vi "Batched Execution Engine constants.vi"() -> ()   [LabVIEW 2010]
uses:
  <vilib>/addons/database/_DB Variant To Data/Database Variant To Data.xnode
  <vilib>/Utility/config.llb/Read Key (String).vi
  <vilib>/addons/database/Connection.llb/DB Tools Open Connec (String).vi
  <vilib>/addons/database/Connection.llb/Conn Execute.vi
  <vilib>/addons/database/Recordset.llb/Rec Destroy - Connection.vi
  <vilib>/addons/database/NI_Database_API.lvlib
  <vilib>/xml/NI_XML.lvlib
  <vilib>/Utility/VariantDataType/VariantType.lvlib
  <vilib>/Utility/config.llb/NI_LVConfig.lvlib
panel:
  out "error out 2":errorcluster
  out "Control Value:Get":variant
  out "error in (no error) 2":errorcluster
  out "submit_time":timestamp
  out "exec_time":timestamp
  in  "Parameter out":T1(array[cluster])
  out "error in (no error)":errorcluster
  out "exp_id":i32
  out "Result: XML Footer":string
  out "Result: XML Header":string
  out "Control TAG":string
  out "Indicator TAG":string
  out "Experiment VI":string
  out "Database":string
  out "CSG 2":csg caption="CSG"
  out "CDB 2":cdb caption="CDB"
  out "CXT 2":cxt caption="CXT"
  out "U 65":u64 caption="U 64"
  out "U 33":u32 caption="U 32"
  out "U 17":u16 caption="U 16"
  out "I 9":i64 caption="I 8"
  out "I 65":i64 caption="I 64"
  out "EXT 2":ext caption="EXT"
  out "I16 2":i16
  out "FXP 2":fxp<+,1,1> caption="FXP"
  out "Single 2":sgl
  out "I 33":i32 caption="I 32"
  out "U 9":i32 caption="U 8"
  out "String 2":string caption="String"
  out "Double 2":dbl caption="Double"
  in  "Parameter in":cluster{"parameter":string, "datatype":string}[](array[cluster])
  out "XML-String-out":string
  in  "input array":variant[](array[variant])
  out "output array":variant[](array[variant])
  out "parse errors":string
  in  "Write Status to Log file":bool
  out "XML-String-in":string
  in  "Stop":bool
  out "Status":string
  # "Parameter Tag"
  # "Parameter data type"
  # "Result Tag"
  # "Result Attribute"
  # "Settings"
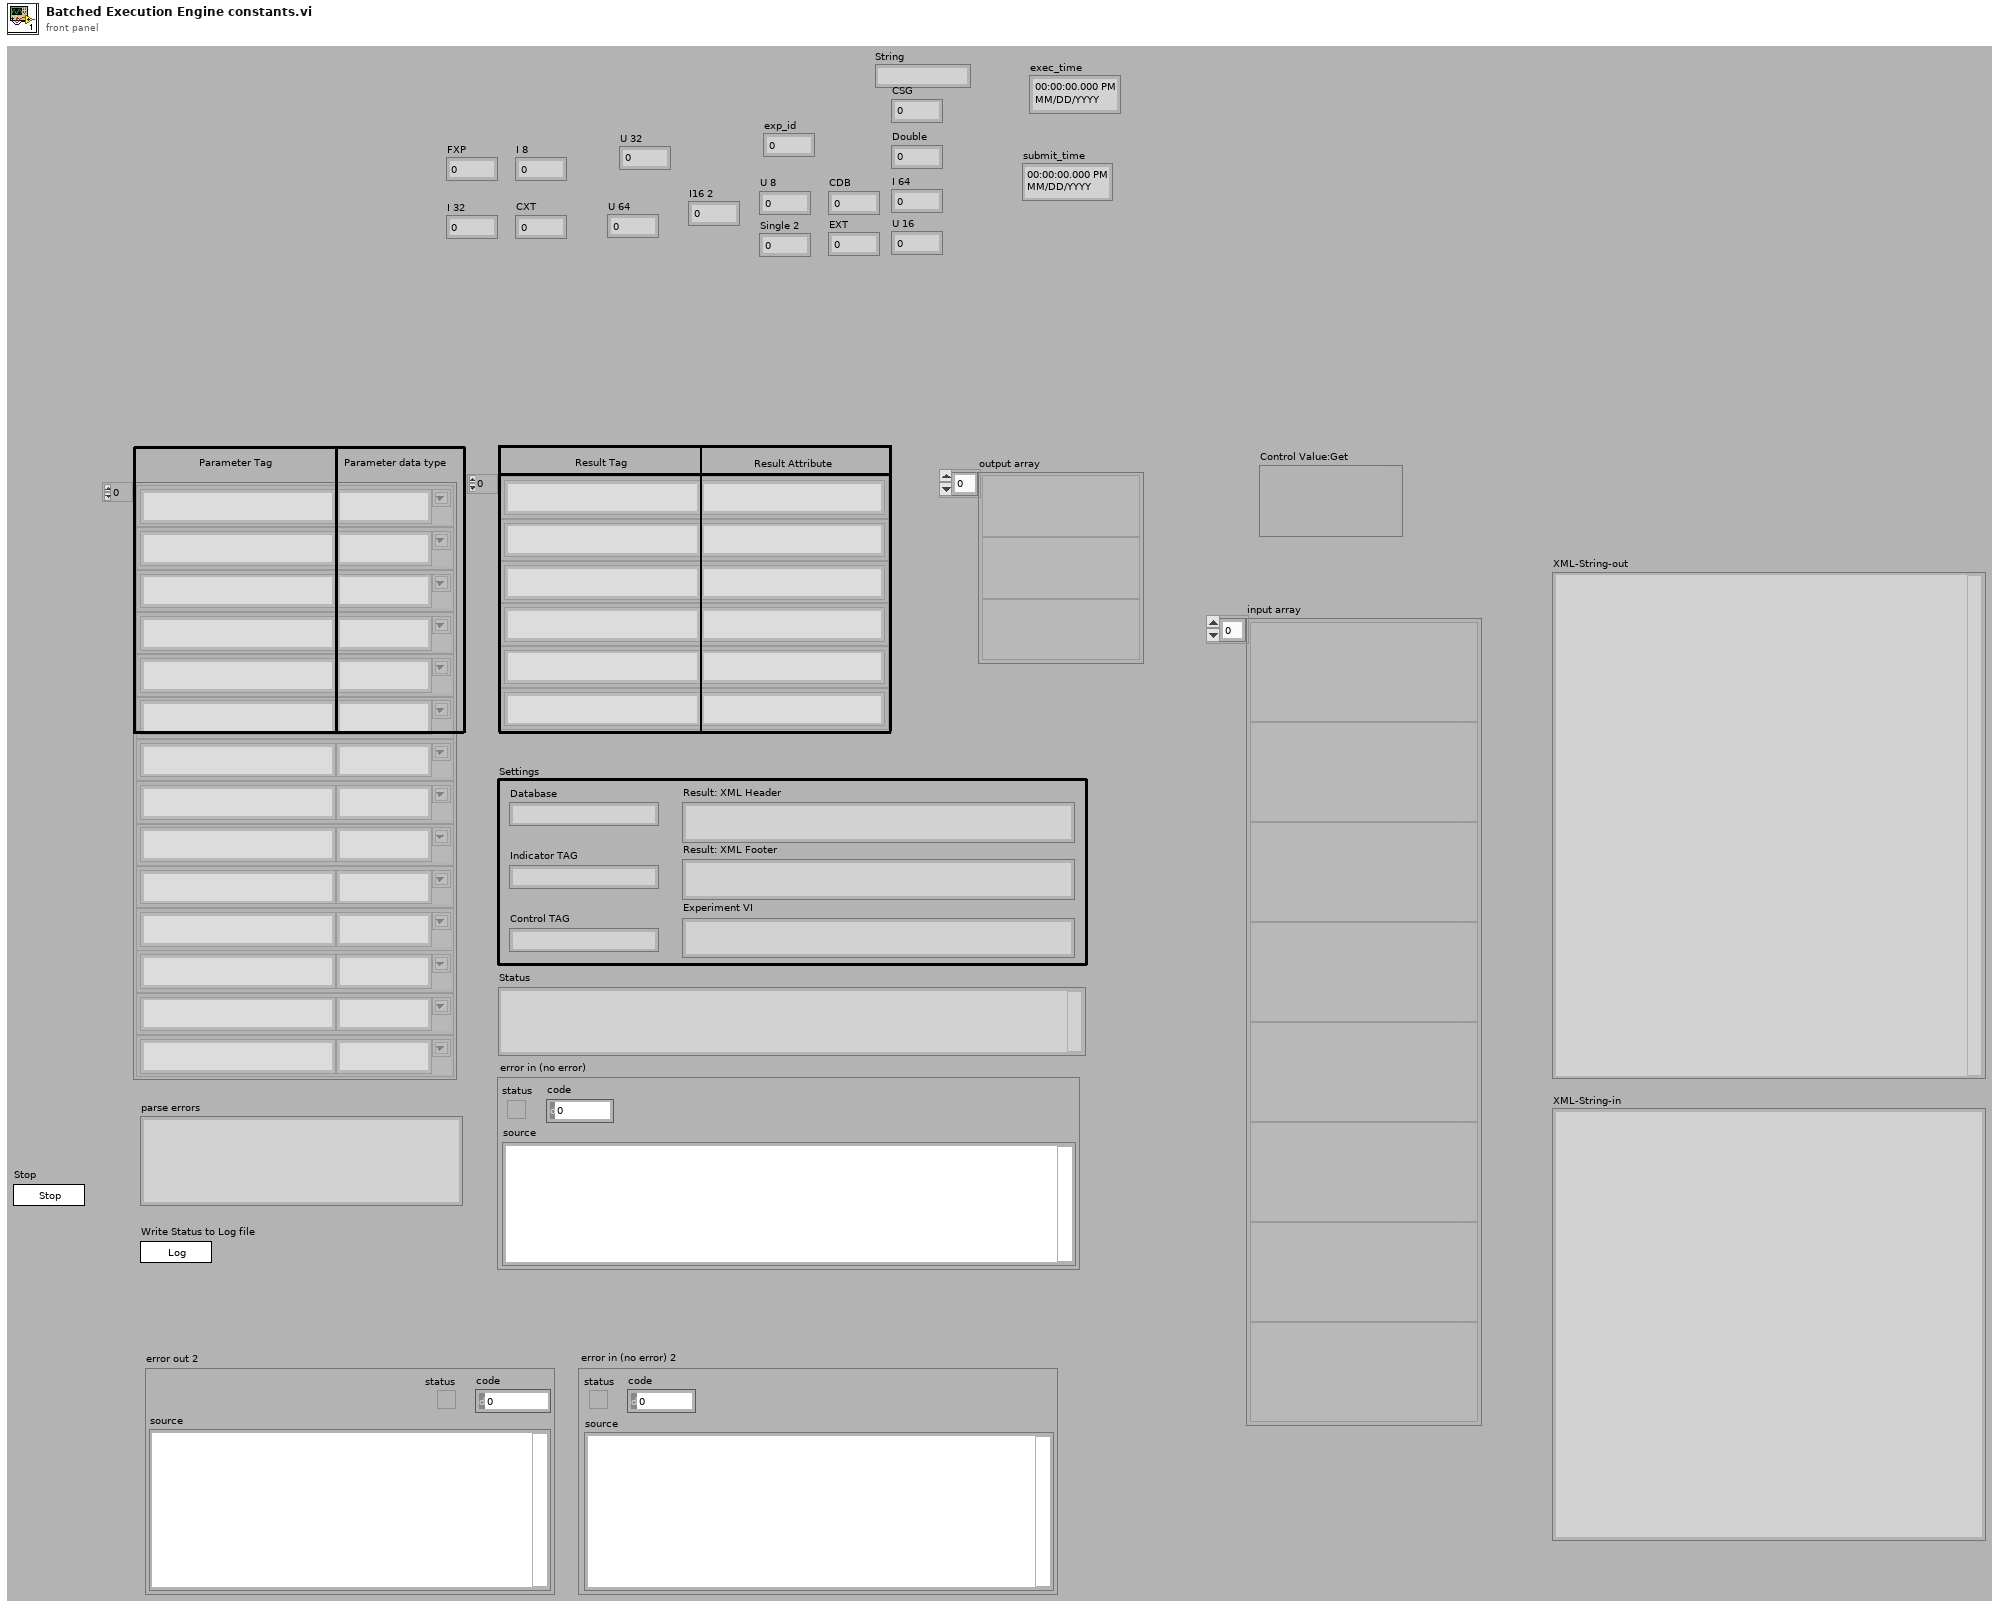
[diagram p1: front panel]
types:
  T1 = cluster{"parameter":string, "type info":string}[]
  T2 = enum16{"Search", "Parse", "Run", "Assemble", "Set", ""}
  T3 = typedef "NI_LVConfig.lvlib/Config Data RefNum.ctl" = refnum<k1>
  T4 = typedef "NI_Database_API.lvlib/Conn ObjectReference.ctl" = refnum<k1>
  T5 = typedef "NI_Database_API.lvlib/Rec ObjectReference.ctl" = refnum<k1>
  T6 = typedef "VariantType.lvlib/Type.ctl" = enum8{"Invalid Type", "Void", "I8", "I16", "I32", "I64", "U8", "U16", "U32", "U64", "Single Float", "Double Float", "Extended Float", "Single Complex", "Double Complex", "Extended Complex", "Enum U8", "Enum U16", "Enum U32", "Enum U64", "Single Float With Unit", "Double Float With Unit", "Extended Float With Unit", "Single Complex with Unit", "Double Complex with Unit", "Extended Complex with Unit", "Boolean", "String", "Path", "Picture", "Tag", "Array", "Cluster", "Variant", "LV Variant", "Waveform", "Timestamp", "Digital Waveform", "Digital Data", "ExpressData", "Refnum", "External Data", "VI", "Poly VI", "LabVIEW Class Instance", "Fixed Point"}
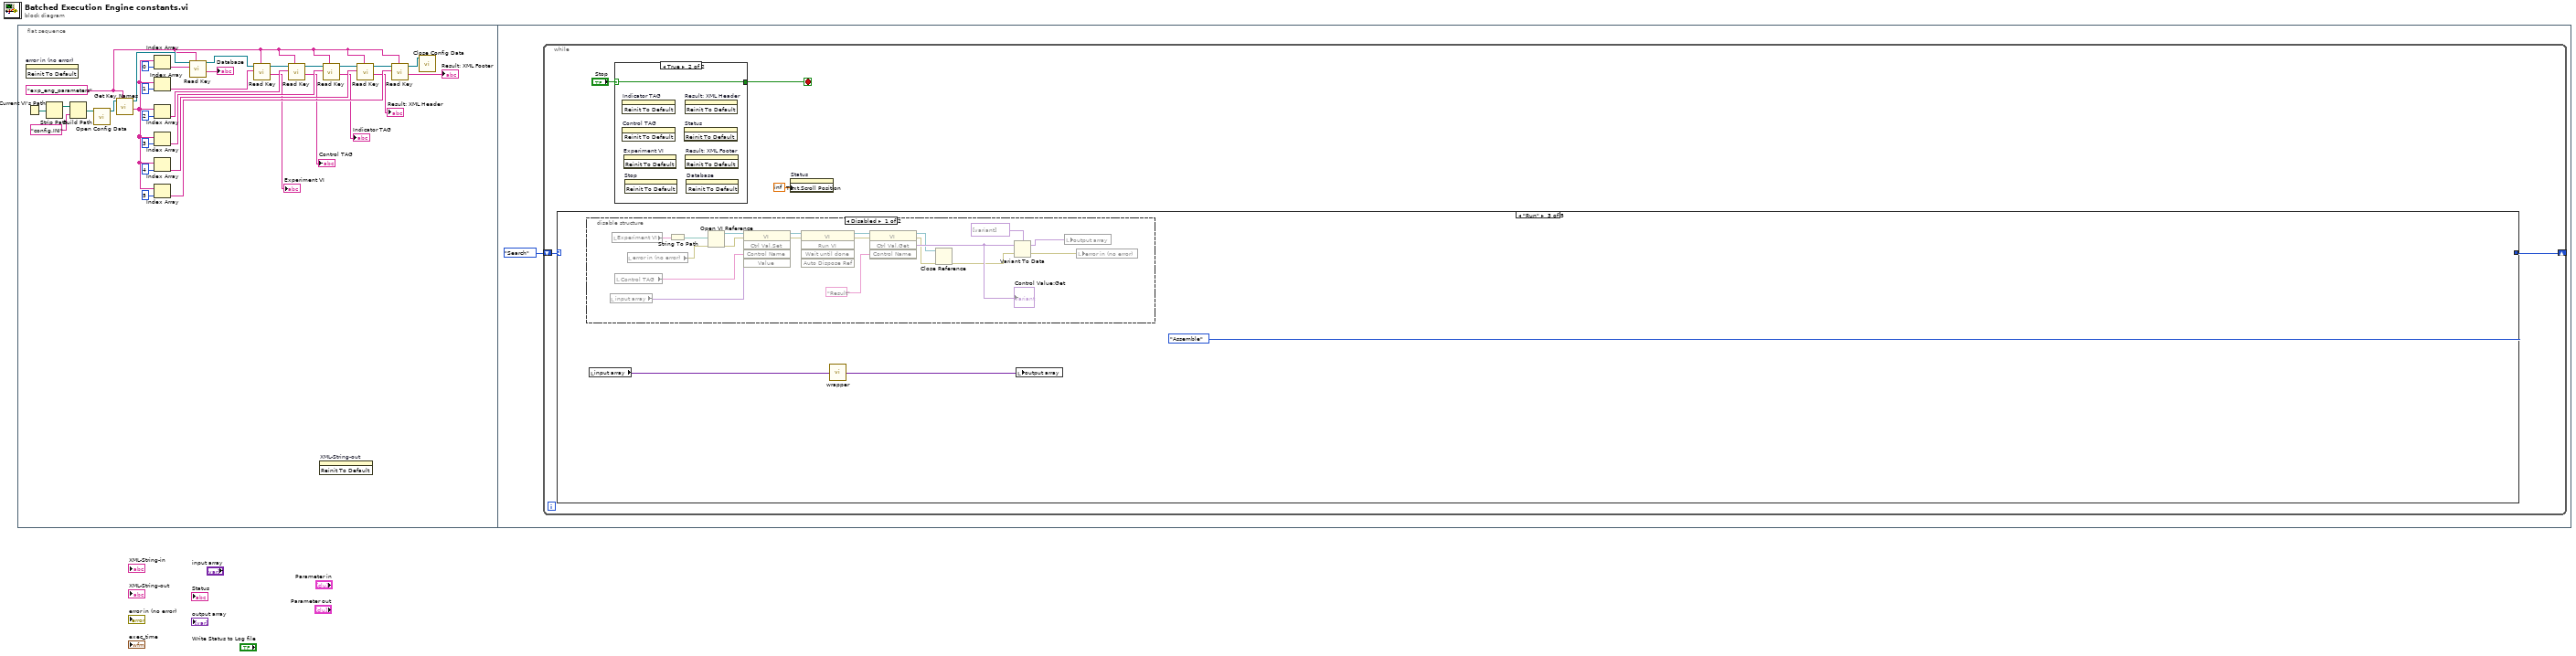
[diagram p0: block diagram]
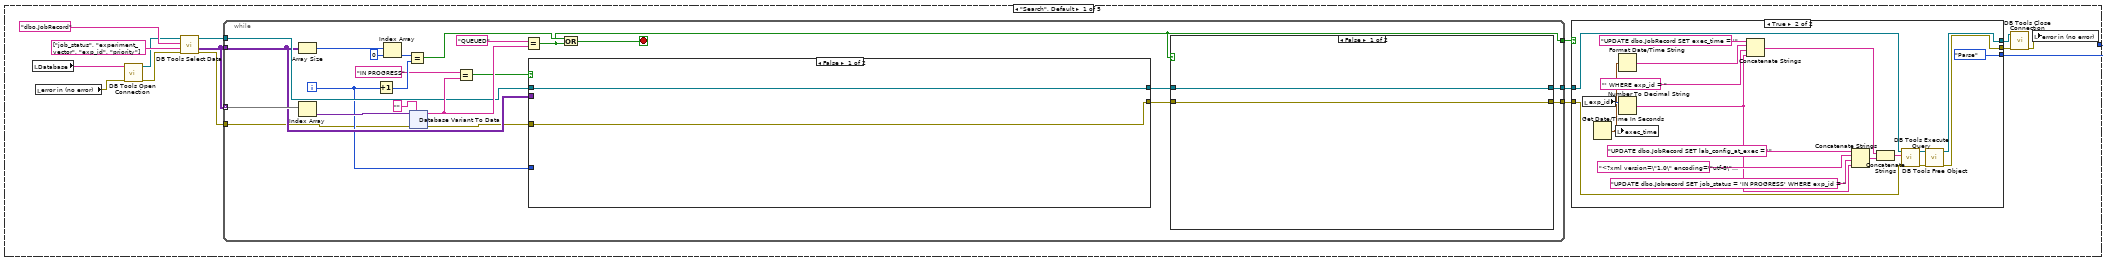
[diagram p3: hidden frame]
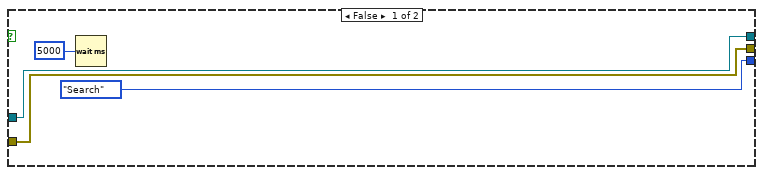
[diagram p4: hidden frame]
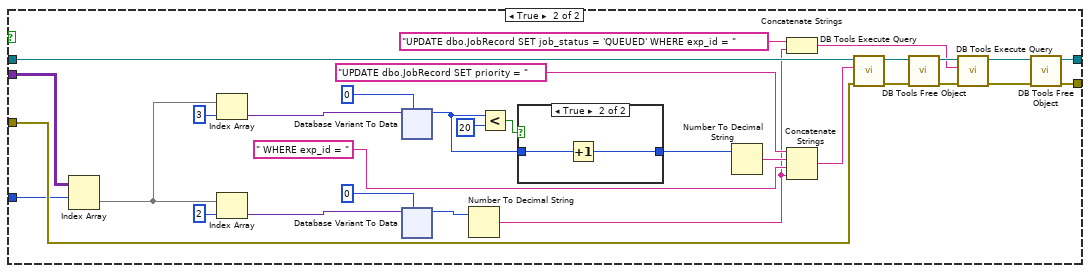
[diagram p5: hidden frame]
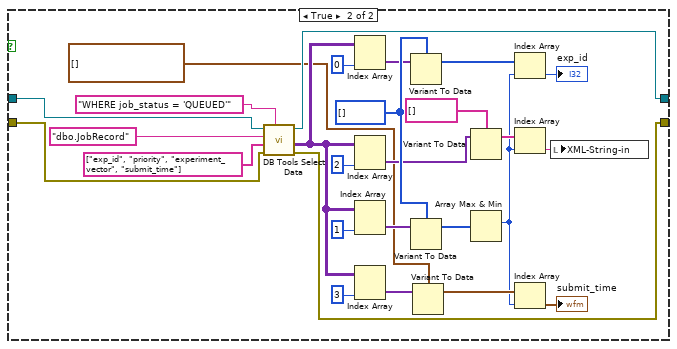
[diagram p7: hidden frame]
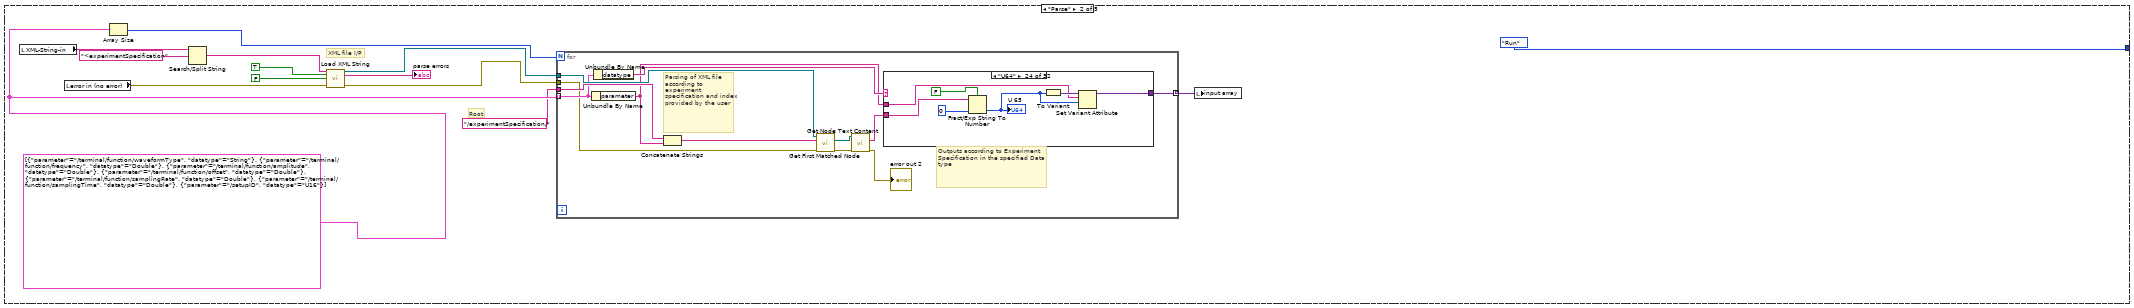
[diagram p8: hidden frame]
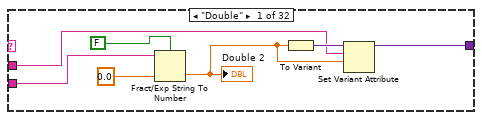
[diagram p9: hidden frame]
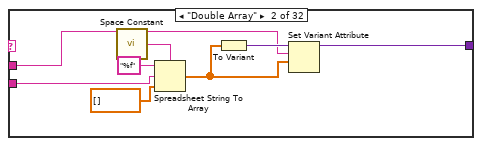
[diagram p10: hidden frame]
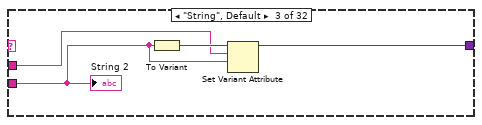
[diagram p11: hidden frame]
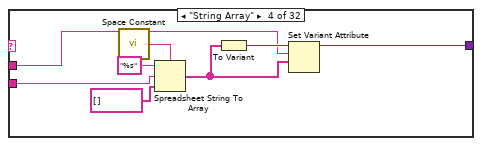
[diagram p12: hidden frame]
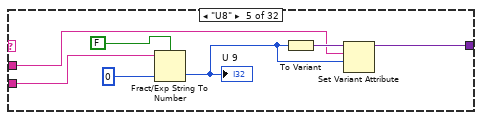
[diagram p13: hidden frame]
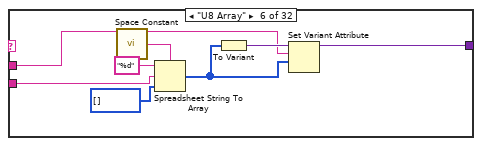
[diagram p14: hidden frame]
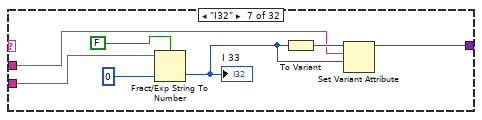
[diagram p15: hidden frame]
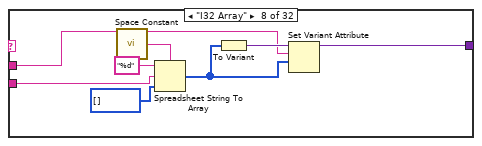
[diagram p16: hidden frame]
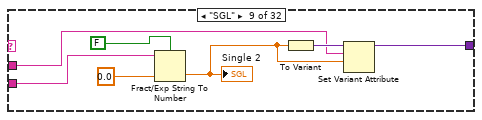
[diagram p17: hidden frame]
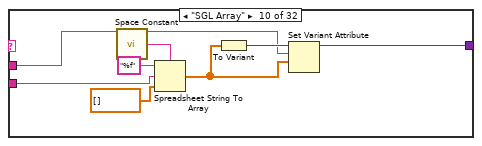
[diagram p18: hidden frame]
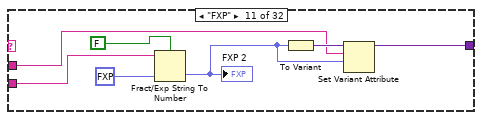
[diagram p19: hidden frame]
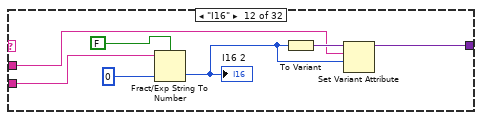
[diagram p20: hidden frame]
diagram:
  n1 = flat-sequence {
    frame #0 {
      w9 = "exp_eng_parameters" ("section")
      n2 = invoke on="error in (no error)" class="Clust (strict)" method="Reinit To Default"() -> ()  [unwired: 3 in, 3 out]
      n3 = Current VI's Path() -> (path=w32:path)
      n4 = Strip Path(path=w32) -> (stripped path=w31:path)  [unwired: 1 out]
      n5 = Build Path(base path=w31, name or relative path="config.INI") -> (appended path=w30:path)
      n6 = call <vilib>:"Open Config Data.vi"("configuration file path"=w30) -> ("refnum"=w28:T3)  [unwired: 8 in, 2 out]
      n7 = call <vilib>:"Get Key Names.vi"("section"=w9, "refnum"=w28) -> ("key names"=w11:string[], "refnum out"=w27:T3)  [unwired: 6 in, 2 out]
      n8 = Index Array(array=w11, index=0) -> (element=w25:string)
      n9 = Index Array(array=w11, index=1) -> (element=w23:string)
      n10 = Index Array(array=w11, index=2) -> (element=w19:string)
      n11 = Index Array(array=w11, index=3) -> (element=w16:string)
      n12 = Index Array(array=w11, index=4) -> (element=w14:string)
      n13 = Index Array(array=w11, index=5) -> (element=w10:string)
      n14 = call-poly <vilib>:"Read Key.vi"("section"=w9, "key"=w25, "refnum"=w27) -> ("value"=→"Database":string, "refnum out"=w22:T3)  [unwired: 5 in, 2 out]
      n15 = call-poly <vilib>:"Read Key.vi"("section"=w9, "key"=w23, "refnum"=w22) -> ("value"=→"Experiment VI":string, "refnum out"=w20:T3)  [unwired: 5 in, 2 out]
      n16 = call-poly <vilib>:"Read Key.vi"("section"=w9, "key"=w19, "refnum"=w20) -> ("value"=→"Control TAG":string, "refnum out"=w17:T3)  [unwired: 5 in, 2 out]
      n17 = invoke on="XML-String-out" class="Str" method="Reinit To Default"() -> ()  [unwired: 3 in, 3 out]
      n18 = call-poly <vilib>:"Read Key.vi"("section"=w9, "key"=w16, "refnum"=w17) -> ("value"=→"Indicator TAG":string, "refnum out"=w13:T3)  [unwired: 5 in, 2 out]
      n19 = call-poly <vilib>:"Read Key.vi"("section"=w9, "key"=w14, "refnum"=w13) -> ("value"=→"Result: XML Header":string, "refnum out"=w8:T3)  [unwired: 5 in, 2 out]
      n20 = call-poly <vilib>:"Read Key.vi"("section"=w9, "key"=w10, "refnum"=w8) -> ("value"=→"Result: XML Footer":string, "refnum out"=w7:T3)  [unwired: 5 in, 2 out]
      n21 = call <vilib>:"Close Config Data.vi"("refnum"=w7) -> ()  [unwired: 9 in, 2 out]
    }
    frame #1 {
      n22 = while {
        shift-right: [w37] -> _
        shift-left: T2."Search" -> [w38]
        stop <- w34 stop-if-true
        n23 = case shown="\"Run\"" w38 {
          tunnel: [w52 T2."Run" T2."Assemble" T2."Set" T2."Search"] -> w37
          frame "Search", Default {
            n24 = local read "Database"() -> (w51:string)
            n25 = local read "error in (no error)"() -> (w47:errorcluster)
            n26 = call-poly <vilib>:"DB Tools Open Connection.vi"("error in (no error)"=w47, "connection information"=w51) -> ("error out"=w54:errorcluster, "connection reference"=w42:T4)  [unwired: 6 in]
            n27 = call <vilib>:"DB Tools Select Data.vi"("error in (no error)"=w54, "columns"=string[] ["job_status", "experiment_vector", "exp_id", "priority"], "table"="dbo.JobRecord", "connection reference"=w42) -> ("error out"=w46:errorcluster, "data"=w53:variant[][], "connection reference out"=w41:T4)  [unwired: 2 in]
            n28 = while {
              tunnel: w41 -> [w90]
              tunnel: [w94] -> w50
              tunnel: w53 -> [w99] mode=indexing
              tunnel: w53 -> [w88]
              tunnel: [w85] -> w43
              tunnel: w46 -> [w81]
              tunnel: [w82] -> w45
              i -> [w87]
              stop <- w84 stop-if-true
              n29 = Array Size(array=w88) -> (size(s)=w98:i32[])
              n30 = Index Array(array=w99) -> (element=w100:variant)  [unwired: 1 in]
              n31 = Increment(x=w87) -> (x+1=w95:i32)
              n32 = Index Array(array=w98, index=0) -> (element=w96:i32)
              n33 = Equal?(x=w96, y=w95) -> (x = y?=w86:bool)
              n34 = xnode "Database Variant To Data"("database variant"=w100, "error in"=w81, "type"="") -> ("data"=w93:string, "error out"=w80:errorcluster)
              n35 = Equal?(x="IN PROGRESS", y=w93) -> (x = y?=w91:bool)
              n36 = Equal?(x="QUEUED", y=w93) -> (x = y?=w85:bool)
              n37 = case shown="False" w91 {
                tunnel: w90 -> [w104 w124]
                tunnel: [w104 w120] -> w89
                tunnel: w88 -> [_ w135]
                tunnel: w87 -> [_ w105]
                tunnel: w80 -> [w103 w111]
                tunnel: [w103 w107] -> w83
                frame False {
                }
                frame True {
                  n38 = Index Array(array=w135, index (row)=w105) -> (element=w128:variant[])  [unwired: 1 in]
                  n39 = Index Array(array=w128, index=3) -> (element=w133:variant)
                  n40 = Index Array(array=w128, index=2) -> (element=w126:variant)
                  n41 = xnode "Database Variant To Data"("database variant"=w133, "type"=0 ("index")) -> ("data"=w129:i32)  [unwired: 1 in, 1 out]
                  n42 = xnode "Database Variant To Data"("database variant"=w126, "type"=0 ("index")) -> ("data"=w115:i32)  [unwired: 1 in, 1 out]
                  n43 = Number To Decimal String(number=w115) -> (decimal integer string=w112:string)  [unwired: 1 in]
                  n44 = Less?(x=w129, y=20) -> (x < y?=w130:bool)
                  n45 = case shown="True" w130 {
                    tunnel: w129 -> [w168 w170]
                    tunnel: [w168 w169] -> w118
                    frame False {
                    }
                    frame True {
                      n46 = Increment(x=w170) -> (x+1=w169:i32)
                    }
                  }
                  n47 = Number To Decimal String(number=w118) -> (decimal integer string=w117:string)  [unwired: 1 in]
                  n48 = Concatenate Strings("UPDATE dbo.JobRecord SET job_status = 'QUEUED' WHERE exp_id = " ("string"), w112) -> (w106:string)
                  n49 = Concatenate Strings("UPDATE dbo.JobRecord SET priority = " ("string"), w117, " WHERE exp_id = " ("string"), w112) -> (w114:string)
                  n50 = call-poly <vilib>:"DB Tools Execute Query.vi"("error in (no error)"=w111, "SQL query"=w114, "connection reference"=w124) -> ("error out"=w110:errorcluster, "recordset reference"=w123:T5)  [unwired: 5 in]
                  n51 = call-poly <vilib>:"DB Tools Free Object.vi"("error in (no error)"=w110, "recordset reference"=w123) -> ("error out"=w109:errorcluster, "connection reference"=w122:T4)  [unwired: 8 in]
                  n52 = call-poly <vilib>:"DB Tools Execute Query.vi"("error in (no error)"=w109, "SQL query"=w106, "connection reference"=w122) -> ("error out"=w108:errorcluster, "recordset reference"=w121:T5)  [unwired: 5 in]
                  n53 = call-poly <vilib>:"DB Tools Free Object.vi"("error in (no error)"=w108, "recordset reference"=w121) -> ("error out"=w107:errorcluster, "connection reference"=w120:T4)  [unwired: 8 in]
                }
              }
              n54 = Or(x=w86, y=w85) -> (x .or. y?=w84:bool)
              n55 = case shown="False" w85 {
                tunnel: w89 -> [w236 w254]
                tunnel: [w236 w253] -> w94
                tunnel: w83 -> [w235 w248]
                tunnel: [w235 w247] -> w82
                frame False {
                }
                frame True {
                  w261 = i32[] [] ("Array")
                  n56 = call <vilib>:"DB Tools Select Data.vi"("condition"="WHERE job_status = 'QUEUED'" ("optional clause"), "error in (no error)"=w248, "columns"=string[] ["exp_id", "priority", "experiment_vector", "submit_time"], "table"="dbo.JobRecord", "connection reference"=w254) -> ("error out"=w247:errorcluster, "data"=w243:variant[][], "connection reference out"=w253:T4)  [unwired: 1 in]
                  n57 = Index Array(array=w243, index (col)=0 ("disabled index (col)")) -> (element=w260:variant[])  [unwired: 1 in]
                  n58 = Index Array(array=w243, index (col)=2 ("index (row)")) -> (element=w251:variant[])  [unwired: 1 in]
                  n59 = Index Array(array=w243, index (col)=1 ("disabled index (col)")) -> (element=w258:variant[])  [unwired: 1 in]
                  n60 = Index Array(array=w243, index (col)=3 ("disabled index (col)")) -> (element=w241:variant[])  [unwired: 1 in]
                  n61 = Variant To Data(Variant=w260, type=w261) -> (data=w263:i32[])  [unwired: 1 in, 1 out]
                  n62 = Variant To Data(Variant=w258, type=w261) -> (data=w262:i32[])  [unwired: 1 in, 1 out]
                  n63 = Variant To Data(Variant=w241, type=timestamp[] [] ("Array")) -> (data=w239:timestamp[])  [unwired: 1 in, 1 out]
                  n64 = Variant To Data(Variant=w251, type=string[] [] ("Array")) -> (data=w250:string[])  [unwired: 1 in, 1 out]
                  n65 = Array Max & Min(array=w262) -> (max index (indices)=w238:i32)  [unwired: 3 out]
                  n66 = Index Array(array=w263, index=w238) -> (element=→"exp_id":i32)
                  n67 = Index Array(array=w250, index=w238) -> (element=w249:string)
                  n68 = Index Array(array=w239, index=w238) -> (element=→"submit_time":timestamp)
                  n69 = local write "XML-String-in"(w249) -> ()
                }
              }
            }
            n70 = case shown="True" w43 {
              tunnel: [T2."Search" T2."Parse"] -> w52
              tunnel: [w60 w72] -> w49
              tunnel: w50 -> [w60 w78]
              tunnel: w45 -> [w59 w77]
              tunnel: [w59 w75] -> w48
              frame False {
                n71 = Wait (ms)(milliseconds to wait=u32 5000 ("millisecond multiple")) -> ()  [unwired: 1 out]
              }
              frame True {
                n72 = local read "exp_id"() -> (w74:i32)
                n73 = Get Date/Time In Seconds() -> (seconds since 1Jan1904=w61:timestamp)
                n74 = local write "exec_time"(w61) -> ()
                n75 = Format Date/Time String(seconds (now)=w61) -> (date/time string=w70:string)  [unwired: 2 in]
                n76 = Number To Decimal String(number=w74) -> (decimal integer string=w65:string)  [unwired: 1 in]
                n77 = Concatenate Strings("UPDATE dbo.JobRecord SET exec_time = '", w70, "' WHERE exp_id = ", w65) -> (w64:string)
                n78 = Concatenate Strings("UPDATE dbo.JobRecord SET lab_config_at_exec = '" ("string"), "<?xml version=\"1.0\" encoding=\"utf-8\" standalone=\"no\" ?><!DOCTYPE labConfiguration SYSTEM \"http://web.mit.edu/weblab/xml/labConfiguration.dtd\"><labConfiguration lab=\"MIT ELVIS Weblab\" specversion=\"0.1\">'" ("string"), "UPDATE dbo.Jobrecord SET job_status = 'IN PROGRESS' WHERE exp_id = " ("string"), w65) -> (w63:string)
                n79 = Concatenate Strings(w64, w63) -> (w62:string)
                n80 = call-poly <vilib>:"DB Tools Execute Query.vi"("error in (no error)"=w77, "SQL query"=w62, "connection reference"=w78) -> ("error out"=w76:errorcluster, "recordset reference"=w73:T5)  [unwired: 5 in]
                n81 = call-poly <vilib>:"DB Tools Free Object.vi"("error in (no error)"=w76, "recordset reference"=w73) -> ("error out"=w75:errorcluster, "connection reference"=w72:T4)  [unwired: 8 in]
              }
            }
            n82 = call <vilib>:"DB Tools Close Connection.vi"("error in (no error)"=w48, "connection reference"=w49) -> ("error out"=w44:errorcluster)  [unwired: 5 in]
            n83 = local write "error in (no error)"(w44) -> ()
          }
          frame "Parse" {
            w265 = cluster{"parameter":string, "datatype":string}[] [{"parameter"="/terminal/function/waveformType", "datatype"="String"}, {"parameter"="/terminal/function/frequency", "datatype"="Double"}, {"parameter"="/terminal/function/amplitude", "datatype"="Double"}, {"parameter"="/terminal/function/offset", "datatype"="Double"}, {"parameter"="/terminal/function/samplingRate", "datatype"="Double"}, {"parameter"="/terminal/function/samplingTime", "datatype"="Double"}, {"parameter"="/setupID", "datatype"="U16"}]
            # "Root"
            # "XML file I/P"
            n84 = local read "XML-String-in"() -> (w270:string)
            n85 = local read "error in (no error)"() -> (w271:errorcluster)
            n86 = Array Size(array=w265) -> (size(s)=w267:i32)
            n87 = Search/Split String(string=w270, search string/char (-)="<experimentSpecification") -> (match + rest of string=w268:string)  [unwired: 1 in, 2 out]
            n88 = call <vilib>:"Load XML String.vi"("XML string"=w268, "process namespaces (False)"=TRUE, "process schema (False)"=FALSE, "error in (no error)"=w271) -> ("DOM document out"=w273:refnum<k20>, "parse errors"=→"parse errors":string, "error out"=w266:errorcluster)  [unwired: 9 out]
            n89 = for {
              N: w267 -> [_]
              tunnel: w273 -> [w289]
              tunnel: "/experimentSpecification/" -> [w287]
              tunnel: w265 -> [w285] mode=indexing
              tunnel: w266 -> [w284]
              tunnel: [w283] -> w272 mode=indexing
              # "Outputs according to Experiment Specification in the specified Data type"
              # "Parsing of XML file according to experiment specification and index provided by the user"
              n90 = Unbundle By Name(w285) -> ("parameter"=w280:string)
              n91 = Unbundle By Name(w285) -> ("datatype"=w282:string)
              n92 = Concatenate Strings(w287, w280) -> (w286:string)
              n93 = call <vilib>:"Get First Matched Node.vi"("error in (no error)"=w284, "XPath expression"=w286, "node in"=w289) -> ("error out"=w278:errorcluster, "node result"=w288:refnum<k20>)  [unwired: 6 in, 1 out]
              n94 = call <vilib>:"Get Node Text Content.vi"("error in (no error)"=w278, "node in"=w288) -> ("error out"=→"error out 2":errorcluster, "node text"=w281:string)  [unwired: 7 in, 1 out]
              n95 = case shown="\"U64\"" w282 {
                tunnel: w280 -> [w290 w298 w305 w309 w317 w324 w332 w340 w347 w355 w362 w369 w376 w384 w392 w399 w406 w414 w421 w429 w436 w444 w451 w459 w466 w474 w482 w490 w497 w504 w512 w519]
                tunnel: w281 -> [w291 w297 w306 w310 w318 w325 w333 w339 w348 w354 w363 w370 w377 w385 w391 w400 w407 w415 w422 w430 w437 w445 w452 w460 w467 w475 w481 w489 w496 w505 w511 w520]
                tunnel: [w293 w300 w307 w313 w320 w328 w335 w343 w350 w357 w365 w372 w380 w387 w394 w402 w410 w417 w425 w432 w440 w447 w455 w462 w470 w477 w484 w492 w499 w507 w514 w522] -> w283
                frame "Double" {
                  n96 = Fract/Exp String To Number(use system decimal point (T)=FALSE, string=w291, default (0 dbl)=0.0) -> (number=w292:dbl)  [unwired: 1 in, 1 out]
                  "Double 2" <- w292
                  n97 = To Variant(anything=w292) -> (Variant=w294:variant)
                  n98 = Set Variant Attribute(Variant=w294, name=w290, value=w292) -> (Variant out=w293:variant)  [unwired: 1 in, 2 out]
                }
                frame "Double Array" {
                  n99 = call <vilib>:"Space Constant.vi"() -> ("String"=w302:string)
                  n100 = Spreadsheet String To Array(delimiter (Tab)=w302, format string="%f", spreadsheet string=w297, array type (2D Dbl)=dbl[] [] ("Array")) -> (array=w299:dbl[])
                  n101 = To Variant(anything=w299) -> (Variant=w301:variant)
                  n102 = Set Variant Attribute(Variant=w301, name=w298, value=w299) -> (Variant out=w300:variant)  [unwired: 1 in, 2 out]
                }
                frame "String", Default {
                  n103 = To Variant(anything=w306) -> (Variant=w308:variant)
                  n104 = Set Variant Attribute(Variant=w308, name=w305, value=w306) -> (Variant out=w307:variant)  [unwired: 1 in, 2 out]
                  "String 2" <- w306
                }
                frame "String Array" {
                  n105 = call <vilib>:"Space Constant.vi"() -> ("String"=w315:string)
                  n106 = Spreadsheet String To Array(delimiter (Tab)=w315, format string="%s", spreadsheet string=w310, array type (2D Dbl)=string[] [] ("Array")) -> (array=w312:string[])
                  n107 = To Variant(anything=w312) -> (Variant=w314:variant)
                  n108 = Set Variant Attribute(Variant=w314, name=w309, value=w312) -> (Variant out=w313:variant)  [unwired: 1 in, 2 out]
                }
                frame "U8" {
                  n109 = Fract/Exp String To Number(use system decimal point (T)=FALSE, string=w318, default (0 dbl)=u8 0) -> (number=w319:u8)  [unwired: 1 in, 1 out]
                  "U 9" <- w319
                  n110 = To Variant(anything=w319) -> (Variant=w321:variant)
                  n111 = Set Variant Attribute(Variant=w321, name=w317, value=w319) -> (Variant out=w320:variant)  [unwired: 1 in, 2 out]
                }
                frame "U8 Array" {
                  n112 = call <vilib>:"Space Constant.vi"() -> ("String"=w330:string)
                  n113 = Spreadsheet String To Array(delimiter (Tab)=w330, format string="%d", spreadsheet string=w325, array type (2D Dbl)=u8[] [] ("Array")) -> (array=w326:u8[])
                  n114 = To Variant(anything=w326) -> (Variant=w329:variant)
                  n115 = Set Variant Attribute(Variant=w329, name=w324, value=w326) -> (Variant out=w328:variant)  [unwired: 1 in, 2 out]
                }
                frame "I32" {
                  n116 = Fract/Exp String To Number(use system decimal point (T)=FALSE, string=w333, default (0 dbl)=0) -> (number=w334:i32)  [unwired: 1 in, 1 out]
                  "I 33" <- w334
                  n117 = To Variant(anything=w334) -> (Variant=w336:variant)
                  n118 = Set Variant Attribute(Variant=w336, name=w332, value=w334) -> (Variant out=w335:variant)  [unwired: 1 in, 2 out]
                }
                frame "I32 Array" {
                  n119 = call <vilib>:"Space Constant.vi"() -> ("String"=w345:string)
                  n120 = Spreadsheet String To Array(delimiter (Tab)=w345, format string="%d", spreadsheet string=w339, array type (2D Dbl)=i32[] [] ("Array")) -> (array=w341:i32[])
                  n121 = To Variant(anything=w341) -> (Variant=w344:variant)
                  n122 = Set Variant Attribute(Variant=w344, name=w340, value=w341) -> (Variant out=w343:variant)  [unwired: 1 in, 2 out]
                }
                frame "SGL" {
                  n123 = Fract/Exp String To Number(use system decimal point (T)=FALSE, string=w348, default (0 dbl)=sgl 0.0) -> (number=w349:sgl)  [unwired: 1 in, 1 out]
                  "Single 2" <- w349
                  n124 = To Variant(anything=w349) -> (Variant=w351:variant)
                  n125 = Set Variant Attribute(Variant=w351, name=w347, value=w349) -> (Variant out=w350:variant)  [unwired: 1 in, 2 out]
                }
                frame "SGL Array" {
                  n126 = call <vilib>:"Space Constant.vi"() -> ("String"=w359:string)
                  n127 = Spreadsheet String To Array(delimiter (Tab)=w359, format string="%f", spreadsheet string=w354, array type (2D Dbl)=sgl[] [] ("Array")) -> (array=w356:sgl[])
                  n128 = To Variant(anything=w356) -> (Variant=w358:variant)
                  n129 = Set Variant Attribute(Variant=w358, name=w355, value=w356) -> (Variant out=w357:variant)  [unwired: 1 in, 2 out]
                }
                frame "FXP" {
                  n130 = Fract/Exp String To Number(use system decimal point (T)=FALSE, string=w363, default (0 dbl)=fxp<+,1,1> 0.0) -> (number=w364:fxp<+,1,1>)  [unwired: 1 in, 1 out]
                  "FXP 2" <- w364
                  n131 = To Variant(anything=w364) -> (Variant=w366:variant)
                  n132 = Set Variant Attribute(Variant=w366, name=w362, value=w364) -> (Variant out=w365:variant)  [unwired: 1 in, 2 out]
                }
                frame "I16" {
                  n133 = Fract/Exp String To Number(use system decimal point (T)=FALSE, string=w370, default (0 dbl)=i16 0 ("I16")) -> (number=w373:i16)  [unwired: 1 in, 1 out]
                  "I16 2" <- w373
                  n134 = To Variant(anything=w373) -> (Variant=w374:variant)
                  n135 = Set Variant Attribute(Variant=w374, name=w369, value=w373) -> (Variant out=w372:variant)  [unwired: 1 in, 2 out]
                }
                frame "I16 Array" {
                  n136 = call <vilib>:"Space Constant.vi"() -> ("String"=w382:string)
                  n137 = Spreadsheet String To Array(delimiter (Tab)=w382, format string="%d", spreadsheet string=w377, array type (2D Dbl)=i16[] [] ("Array")) -> (array=w378:i16[])
                  n138 = To Variant(anything=w378) -> (Variant=w381:variant)
                  n139 = Set Variant Attribute(Variant=w381, name=w376, value=w378) -> (Variant out=w380:variant)  [unwired: 1 in, 2 out]
                }
                frame "EXT" {
                  n140 = Fract/Exp String To Number(use system decimal point (T)=FALSE, string=w385, default (0 dbl)=ext 0.0) -> (number=w386:ext)  [unwired: 1 in, 1 out]
                  "EXT 2" <- w386
                  n141 = To Variant(anything=w386) -> (Variant=w388:variant)
                  n142 = Set Variant Attribute(Variant=w388, name=w384, value=w386) -> (Variant out=w387:variant)  [unwired: 1 in, 2 out]
                }
                frame "EXT Array" {
                  n143 = call <vilib>:"Space Constant.vi"() -> ("String"=w396:string)
                  n144 = Spreadsheet String To Array(delimiter (Tab)=w396, format string="%f", spreadsheet string=w391, array type (2D Dbl)=ext[] [] ("Array")) -> (array=w393:ext[])
                  n145 = To Variant(anything=w393) -> (Variant=w395:variant)
                  n146 = Set Variant Attribute(Variant=w395, name=w392, value=w393) -> (Variant out=w394:variant)  [unwired: 1 in, 2 out]
                }
                frame "I64" {
                  n147 = Fract/Exp String To Number(use system decimal point (T)=FALSE, string=w400, default (0 dbl)=i64 0) -> (number=w401:i64)  [unwired: 1 in, 1 out]
                  "I 65" <- w401
                  n148 = To Variant(anything=w401) -> (Variant=w403:variant)
                  n149 = Set Variant Attribute(Variant=w403, name=w399, value=w401) -> (Variant out=w402:variant)  [unwired: 1 in, 2 out]
                }
                frame "I64 Array" {
                  n150 = call <vilib>:"Space Constant.vi"() -> ("String"=w412:string)
                  n151 = Spreadsheet String To Array(delimiter (Tab)=w412, format string="%d", spreadsheet string=w407, array type (2D Dbl)=i64[] [] ("Array")) -> (array=w408:i64[])
                  n152 = To Variant(anything=w408) -> (Variant=w411:variant)
                  n153 = Set Variant Attribute(Variant=w411, name=w406, value=w408) -> (Variant out=w410:variant)  [unwired: 1 in, 2 out]
                }
                frame "I8" {
                  n154 = Fract/Exp String To Number(use system decimal point (T)=FALSE, string=w415, default (0 dbl)=i8 0) -> (number=w416:i8)  [unwired: 1 in, 1 out]
                  "I 9" <- w416
                  n155 = To Variant(anything=w416) -> (Variant=w418:variant)
                  n156 = Set Variant Attribute(Variant=w418, name=w414, value=w416) -> (Variant out=w417:variant)  [unwired: 1 in, 2 out]
                }
                frame "I8 Array" {
                  n157 = call <vilib>:"Space Constant.vi"() -> ("String"=w427:string)
                  n158 = Spreadsheet String To Array(delimiter (Tab)=w427, format string="%d", spreadsheet string=w422, array type (2D Dbl)=i8[] [] ("Array")) -> (array=w423:i8[])
                  n159 = To Variant(anything=w423) -> (Variant=w426:variant)
                  n160 = Set Variant Attribute(Variant=w426, name=w421, value=w423) -> (Variant out=w425:variant)  [unwired: 1 in, 2 out]
                }
                frame "U16" {
                  n161 = Fract/Exp String To Number(use system decimal point (T)=FALSE, string=w430, default (0 dbl)=u16 0) -> (number=w431:u16)  [unwired: 1 in, 1 out]
                  "U 17" <- w431
                  n162 = To Variant(anything=w431) -> (Variant=w433:variant)
                  n163 = Set Variant Attribute(Variant=w433, name=w429, value=w431) -> (Variant out=w432:variant)  [unwired: 1 in, 2 out]
                }
                frame "U16 Array" {
                  n164 = call <vilib>:"Space Constant.vi"() -> ("String"=w442:string)
                  n165 = Spreadsheet String To Array(delimiter (Tab)=w442, format string="%d", spreadsheet string=w437, array type (2D Dbl)=u16[] [] ("Array")) -> (array=w438:u16[])
                  n166 = To Variant(anything=w438) -> (Variant=w441:variant)
                  n167 = Set Variant Attribute(Variant=w441, name=w436, value=w438) -> (Variant out=w440:variant)  [unwired: 1 in, 2 out]
                }
                frame "U32" {
                  n168 = Fract/Exp String To Number(use system decimal point (T)=FALSE, string=w445, default (0 dbl)=u32 0) -> (number=w446:u32)  [unwired: 1 in, 1 out]
                  "U 33" <- w446
                  n169 = To Variant(anything=w446) -> (Variant=w448:variant)
                  n170 = Set Variant Attribute(Variant=w448, name=w444, value=w446) -> (Variant out=w447:variant)  [unwired: 1 in, 2 out]
                }
                frame "U32 Array" {
                  n171 = call <vilib>:"Space Constant.vi"() -> ("String"=w457:string)
                  n172 = Spreadsheet String To Array(delimiter (Tab)=w457, format string="%d", spreadsheet string=w452, array type (2D Dbl)=u32[] [] ("Array")) -> (array=w453:u32[])
                  n173 = To Variant(anything=w453) -> (Variant=w456:variant)
                  n174 = Set Variant Attribute(Variant=w456, name=w451, value=w453) -> (Variant out=w455:variant)  [unwired: 1 in, 2 out]
                }
                frame "U64" {
                  n175 = Fract/Exp String To Number(use system decimal point (T)=FALSE, string=w460, default (0 dbl)=u64 0) -> (number=w461:u64)  [unwired: 1 in, 1 out]
                  "U 65" <- w461
                  n176 = To Variant(anything=w461) -> (Variant=w463:variant)
                  n177 = Set Variant Attribute(Variant=w463, name=w459, value=w461) -> (Variant out=w462:variant)  [unwired: 1 in, 2 out]
                }
                frame "U64 Array" {
                  n178 = call <vilib>:"Space Constant.vi"() -> ("String"=w472:string)
                  n179 = Spreadsheet String To Array(delimiter (Tab)=w472, format string="%d", spreadsheet string=w467, array type (2D Dbl)=u64[] [] ("Array")) -> (array=w468:u64[])
                  n180 = To Variant(anything=w468) -> (Variant=w471:variant)
                  n181 = Set Variant Attribute(Variant=w471, name=w466, value=w468) -> (Variant out=w470:variant)  [unwired: 1 in, 2 out]
                }
                frame "CXT" {
                  n182 = Scan From String(format string="%f", input string=w475, default 1=cxt 0.0+0.0i ("number 3")) -> (output 1=w476:cxt)  [unwired: 2 in, 3 out]
                  "CXT 2" <- w476
                  n183 = To Variant(anything=w476) -> (Variant=w478:variant)
                  n184 = Set Variant Attribute(Variant=w478, name=w474, value=w476) -> (Variant out=w477:variant)  [unwired: 1 in, 2 out]
                }
                frame "CXT Array" {
                  n185 = call <vilib>:"Space Constant.vi"() -> ("String"=w486:string)
                  n186 = Spreadsheet String To Array(delimiter (Tab)=w486, format string="%f", spreadsheet string=w481, array type (2D Dbl)=cxt[] [] ("Array")) -> (array=w483:cxt[])
                  n187 = To Variant(anything=w483) -> (Variant=w485:variant)
                  n188 = Set Variant Attribute(Variant=w485, name=w482, value=w483) -> (Variant out=w484:variant)  [unwired: 1 in, 2 out]
                }
                frame "CDB" {
                  n189 = Scan From String(format string="%f", input string=w489, default 1=cdb 0.0+0.0i ("number 3")) -> (output 1=w491:cdb)  [unwired: 2 in, 3 out]
                  "CDB 2" <- w491
                  n190 = To Variant(anything=w491) -> (Variant=w493:variant)
                  n191 = Set Variant Attribute(Variant=w493, name=w490, value=w491) -> (Variant out=w492:variant)  [unwired: 1 in, 2 out]
                }
                frame "CDB Array" {
                  n192 = call <vilib>:"Space Constant.vi"() -> ("String"=w501:string)
                  n193 = Spreadsheet String To Array(delimiter (Tab)=w501, format string="%f", spreadsheet string=w496, array type (2D Dbl)=cdb[] [] ("Array")) -> (array=w498:cdb[])
                  n194 = To Variant(anything=w498) -> (Variant=w500:variant)
                  n195 = Set Variant Attribute(Variant=w500, name=w497, value=w498) -> (Variant out=w499:variant)  [unwired: 1 in, 2 out]
                }
                frame "CSG" {
                  n196 = Scan From String(format string="%f", input string=w505, default 1=csg 0.0+0.0i ("number 3")) -> (output 1=w506:csg)  [unwired: 2 in, 3 out]
                  "CSG 2" <- w506
                  n197 = To Variant(anything=w506) -> (Variant=w508:variant)
                  n198 = Set Variant Attribute(Variant=w508, name=w504, value=w506) -> (Variant out=w507:variant)  [unwired: 1 in, 2 out]
                }
                frame "CSG Array" {
                  n199 = call <vilib>:"Space Constant.vi"() -> ("String"=w516:string)
                  n200 = Spreadsheet String To Array(delimiter (Tab)=w516, format string="%f", spreadsheet string=w511, array type (2D Dbl)=csg[] [] ("Array")) -> (array=w513:csg[])
                  n201 = To Variant(anything=w513) -> (Variant=w515:variant)
                  n202 = Set Variant Attribute(Variant=w515, name=w512, value=w513) -> (Variant out=w514:variant)  [unwired: 1 in, 2 out]
                }
                frame "Boolean" {
                  n203 = case shown="\"False\", Default" w520 {
                    tunnel: [FALSE TRUE TRUE FALSE TRUE FALSE TRUE FALSE] -> w521
                    frame "False", Default {
                    }
                    frame "True" {
                    }
                    frame "TRUE" {
                    }
                    frame "FALSE" {
                    }
                    frame "1" {
                    }
                    frame "0" {
                    }
                    frame "true" {
                    }
                    frame "false" {
                    }
                  }
                  n204 = To Variant(anything=w521) -> (Variant=w523:variant)
                  n205 = Set Variant Attribute(Variant=w523, name=w519, value=w521) -> (Variant out=w522:variant)  [unwired: 1 in, 2 out]
                }
              }
            }
            n206 = local write "input array"(w272) -> ()
          }
          frame "Run" {
            n207 = disable-structure shown="Disabled" {
              frame Disabled {
                n208 = local read "input array"() -> (w536:variant[])
                n209 = local read "Experiment VI"() -> (w547:string)
                n210 = local read "Control TAG"() -> (w548:string)
                n211 = local read "error in (no error)"() -> (w544:errorcluster)
                n212 = String To Path(string=w547) -> (path=w546:path)
                n213 = Open VI Reference(vi path=w546, error in (no error)=w544) -> (vi reference=w553:refnum<vi>, error out=w543:errorcluster)  [unwired: 4 in]
                n214 = invoke class="VI" method="Ctrl Val.Set"(reference=w553, error in=w543, "Control Name"=w548, "Value"=w536) -> (reference out=w549:refnum<vi>, error out=w542:errorcluster)  [unwired: 1 in, 3 out]
                n215 = invoke class="VI" method="Run VI"(reference=w549, error in=w542) -> (reference out=w552:refnum<vi>, error out=w541:errorcluster)  [unwired: 3 in, 3 out]
                n216 = invoke class="VI" method="Ctrl Val.Get"(reference=w552, error in=w541, "Control Name"="Result") -> (reference out=w550:refnum<vi>, error out=w540:errorcluster, "Get Control Value Variant"=w551:variant)  [unwired: 1 in, 1 out]
                "Control Value:Get" <- w551
                n217 = Close Reference(reference=w550, error in (no error)=w540) -> (error out=w539:errorcluster)
                n218 = Variant To Data(error in=w539, Variant=w551, type=variant[] [variant(variant[] [variant(dbl[] array[3004 elements])])] ("output array")) -> (error out=w538:errorcluster, data=w535:variant[])
                n219 = local write "output array"(w535) -> ()
                n220 = local write "error in (no error)"(w538) -> ()
              }
              frame Enabled {
              }
            }
            n221 = local read "input array"() -> (w533:variant[])
            n222 = call "wrapper.vi"("Parameter"=w533) -> ("Result"=w532:variant[])
            n223 = local write "output array"(w532) -> ()
          }
          frame "Assemble" {
            w554 = T1 [{"parameter"="datavector", "type info"="name=''TIME''"}, {"parameter"="datavector", "type info"="name=''VOUT''"}, {"parameter"="datavector", "type info"="name=''VIN''"}] ("Parameter out 2")
            n224 = local read "output array"() -> (w557:variant[])
            n225 = local read "Result: XML Header"() -> (w556:string)
            n226 = local read "Result: XML Footer"() -> (w555:string)
            n227 = Array Size(array=w554) -> (size(s)=w560:i32)
            n228 = for {
              N: w560 -> [_]
              tunnel: w557 -> [w565] mode=indexing
              tunnel: w554 -> [w563] mode=indexing
              tunnel: [w567] -> w558 mode=indexing
              n229 = Unbundle By Name(w563) -> ("parameter"=w566:string)
              n230 = call <vilib>:"GetTypeInfo.vi"("Variant"=w565) -> ("Type Enum"=w564:T6)  [unwired: 6 in, 4 out]
              n231 = Unbundle By Name(w563) -> ("type info"=w562:string)
              n232 = case shown="\"Array\"" w564 {
                tunnel: w566 -> [w569 w593 w618 w641 w666 w689 w713 w737 w761 w786 w811 w836 w860 w884 w908 w933 w1202 w1222]
                tunnel: [w568 w592 w616 w640 w665 w688 w712 w736 w760 w785 w810 w835 w859 w883 w907 w937 w1198 w1221] -> w567
                tunnel: w565 -> [w574 w598 w622 w646 w670 w694 w718 w742 w768 w793 w818 w841 w865 w889 w913 w938 w1204 w1230]
                tunnel: w562 -> [w571 w595 w619 w643 w664 w691 w715 w739 w763 w788 w813 w838 w862 w886 w910 w932 w1200 w1224]
                frame "I8" {
                  n233 = Get Variant Attribute(Variant=w574, name=w569) -> (duplicate Variant=w575:variant)  [unwired: 2 in, 3 out]
                  n234 = Equal?(x=w571, y="") -> (x = y?=w573:bool)
                  n235 = Variant To Data(Variant=w575, type=i8 0) -> (data=w577:i8)  [unwired: 1 in, 1 out]
                  n236 = Number To Decimal String(number=w577) -> (decimal integer string=w570:string)  [unwired: 1 in]
                  n237 = case shown="True" w573 {
                    tunnel: w569 -> [w581 w586]
                    tunnel: w571 -> [w578 _]
                    tunnel: w570 -> [w580 w589]
                    tunnel: [w579 w590] -> w568
                    frame False {
                      w584 = ">" ("string")
                      n238 = call <vilib>:"Space Constant.vi"() -> ("String"=w585:string)
                      n239 = Concatenate Strings("<" ("string"), w581, w585, w578, w584, w580, "</" ("string"), w581, w584) -> (w579:string)
                    }
                    frame True {
                      w587 = ">" ("string")
                      n240 = Concatenate Strings("<" ("string"), w586, w587, w589, "</" ("string"), w586, w587) -> (w590:string)
                    }
                  }
                }
                frame "I16" {
                  n241 = Get Variant Attribute(Variant=w598, name=w593) -> (duplicate Variant=w600:variant)  [unwired: 2 in, 3 out]
                  n242 = Equal?(x=w595, y="") -> (x = y?=w597:bool)
                  n243 = Variant To Data(Variant=w600, type=i16 0 ("I16")) -> (data=w601:i16)  [unwired: 1 in, 1 out]
                  n244 = Number To Decimal String(number=w601) -> (decimal integer string=w594:string)  [unwired: 1 in]
                  n245 = case shown="True" w597 {
                    tunnel: w593 -> [w605 w610]
                    tunnel: w595 -> [w602 _]
                    tunnel: w594 -> [w604 w613]
                    tunnel: [w603 w614] -> w592
                    frame False {
                      w608 = ">" ("string")
                      n246 = call <vilib>:"Space Constant.vi"() -> ("String"=w609:string)
                      n247 = Concatenate Strings("<" ("string"), w605, w609, w602, w608, w604, "</" ("string"), w605, w608) -> (w603:string)
                    }
                    frame True {
                      w611 = ">" ("string")
                      n248 = Concatenate Strings("<" ("string"), w610, w611, w613, "</" ("string"), w610, w611) -> (w614:string)
                    }
                  }
                }
                frame "I32" {
                  n249 = Get Variant Attribute(Variant=w622, name=w618) -> (duplicate Variant=w623:variant)  [unwired: 2 in, 3 out]
                  n250 = Equal?(x=w619, y="") -> (x = y?=w621:bool)
                  n251 = Variant To Data(Variant=w623, type=i16 0 ("precision (6)")) -> (data=w625:i16)  [unwired: 1 in, 1 out]
                  n252 = Number To Decimal String(number=w625) -> (decimal integer string=w617:string)  [unwired: 1 in]
                  n253 = case shown="True" w621 {
                    tunnel: w618 -> [w629 w634]
                    tunnel: w619 -> [w626 _]
                    tunnel: w617 -> [w628 w637]
                    tunnel: [w627 w638] -> w616
                    frame False {
                      w632 = ">" ("string")
                      n254 = call <vilib>:"Space Constant.vi"() -> ("String"=w633:string)
                      n255 = Concatenate Strings("<" ("string"), w629, w633, w626, w632, w628, "</" ("string"), w629, w632) -> (w627:string)
                    }
                    frame True {
                      w635 = ">" ("string")
                      n256 = Concatenate Strings("<" ("string"), w634, w635, w637, "</" ("string"), w634, w635) -> (w638:string)
                    }
                  }
                }
                frame "I64" {
                  n257 = Get Variant Attribute(Variant=w646, name=w641) -> (duplicate Variant=w647:variant)  [unwired: 2 in, 3 out]
                  n258 = Equal?(x=w643, y="") -> (x = y?=w645:bool)
                  n259 = Variant To Data(Variant=w647, type=i64 0) -> (data=w649:i64)  [unwired: 1 in, 1 out]
                  n260 = Number To Decimal String(number=w649) -> (decimal integer string=w642:string)  [unwired: 1 in]
                  n261 = case shown="True" w645 {
                    tunnel: w641 -> [w653 w658]
                    tunnel: w643 -> [w650 _]
                    tunnel: w642 -> [w652 w661]
                    tunnel: [w651 w662] -> w640
                    frame False {
                      w656 = ">" ("string")
                      n262 = call <vilib>:"Space Constant.vi"() -> ("String"=w657:string)
                      n263 = Concatenate Strings("<" ("string"), w653, w657, w650, w656, w652, "</" ("string"), w653, w656) -> (w651:string)
                    }
                    frame True {
                      w659 = ">" ("string")
                      n264 = Concatenate Strings("<" ("string"), w658, w659, w661, "</" ("string"), w658, w659) -> (w662:string)
                    }
                  }
                }
                frame "U8" {
                  n265 = Get Variant Attribute(Variant=w670, name=w666) -> (duplicate Variant=w671:variant)  [unwired: 2 in, 3 out]
                  n266 = Equal?(x=w664, y="") -> (x = y?=w669:bool)
                  n267 = Variant To Data(Variant=w671, type=u8 0) -> (data=w673:u8)  [unwired: 1 in, 1 out]
                  n268 = Number To Decimal String(number=w673) -> (decimal integer string=w667:string)  [unwired: 1 in]
                  n269 = case shown="True" w669 {
                    tunnel: w666 -> [w677 w682]
                    tunnel: w664 -> [w674 _]
                    tunnel: w667 -> [w676 w685]
                    tunnel: [w675 w686] -> w665
                    frame False {
                      w680 = ">" ("string")
                      n270 = call <vilib>:"Space Constant.vi"() -> ("String"=w681:string)
                      n271 = Concatenate Strings("<" ("string"), w677, w681, w674, w680, w676, "</" ("string"), w677, w680) -> (w675:string)
                    }
                    frame True {
                      w683 = ">" ("string")
                      n272 = Concatenate Strings("<" ("string"), w682, w683, w685, "</" ("string"), w682, w683) -> (w686:string)
                    }
                  }
                }
                frame "U16" {
                  n273 = Get Variant Attribute(Variant=w694, name=w689) -> (duplicate Variant=w695:variant)  [unwired: 2 in, 3 out]
                  n274 = Equal?(x=w691, y="") -> (x = y?=w693:bool)
                  n275 = Variant To Data(Variant=w695, type=u16 0) -> (data=w697:u16)  [unwired: 1 in, 1 out]
                  n276 = Number To Decimal String(number=w697) -> (decimal integer string=w690:string)  [unwired: 1 in]
                  n277 = case shown="True" w693 {
                    tunnel: w689 -> [w701 w706]
                    tunnel: w691 -> [w698 _]
                    tunnel: w690 -> [w700 w709]
                    tunnel: [w699 w710] -> w688
                    frame False {
                      w704 = ">" ("string")
                      n278 = call <vilib>:"Space Constant.vi"() -> ("String"=w705:string)
                      n279 = Concatenate Strings("<" ("string"), w701, w705, w698, w704, w700, "</" ("string"), w701, w704) -> (w699:string)
                    }
                    frame True {
                      w707 = ">" ("string")
                      n280 = Concatenate Strings("<" ("string"), w706, w707, w709, "</" ("string"), w706, w707) -> (w710:string)
                    }
                  }
                }
                frame "U32" {
                  n281 = Get Variant Attribute(Variant=w718, name=w713) -> (duplicate Variant=w719:variant)  [unwired: 2 in, 3 out]
                  n282 = Equal?(x=w715, y="") -> (x = y?=w717:bool)
                  n283 = Variant To Data(Variant=w719, type=u32 0) -> (data=w721:u32)  [unwired: 1 in, 1 out]
                  n284 = Number To Decimal String(number=w721) -> (decimal integer string=w714:string)  [unwired: 1 in]
                  n285 = case shown="True" w717 {
                    tunnel: w713 -> [w725 w730]
                    tunnel: w715 -> [w722 _]
                    tunnel: w714 -> [w724 w733]
                    tunnel: [w723 w734] -> w712
                    frame False {
                      w728 = ">" ("string")
                      n286 = call <vilib>:"Space Constant.vi"() -> ("String"=w729:string)
                      n287 = Concatenate Strings("<" ("string"), w725, w729, w722, w728, w724, "</" ("string"), w725, w728) -> (w723:string)
                    }
                    frame True {
                      w731 = ">" ("string")
                      n288 = Concatenate Strings("<" ("string"), w730, w731, w733, "</" ("string"), w730, w731) -> (w734:string)
                    }
                  }
                }
                frame "U64" {
                  n289 = Get Variant Attribute(Variant=w742, name=w737) -> (duplicate Variant=w743:variant)  [unwired: 2 in, 3 out]
                  n290 = Equal?(x=w739, y="") -> (x = y?=w741:bool)
                  n291 = Variant To Data(Variant=w743, type=u64 0) -> (data=w745:u64)  [unwired: 1 in, 1 out]
                  n292 = Number To Decimal String(number=w745) -> (decimal integer string=w738:string)  [unwired: 1 in]
                  n293 = case shown="True" w741 {
                    tunnel: w737 -> [w749 w754]
                    tunnel: w739 -> [w746 _]
                    tunnel: w738 -> [w748 w757]
                    tunnel: [w747 w758] -> w736
                    frame False {
                      w752 = ">" ("string")
                      n294 = call <vilib>:"Space Constant.vi"() -> ("String"=w753:string)
                      n295 = Concatenate Strings("<" ("string"), w749, w753, w746, w752, w748, "</" ("string"), w749, w752) -> (w747:string)
                    }
                    frame True {
                      w755 = ">" ("string")
                      n296 = Concatenate Strings("<" ("string"), w754, w755, w757, "</" ("string"), w754, w755) -> (w758:string)
                    }
                  }
                }
                frame "Single Float" {
                  n297 = Get Variant Attribute(Variant=w768, name=w761) -> (duplicate Variant=w769:variant)  [unwired: 2 in, 3 out]
                  n298 = Equal?(x=w763, y="") -> (x = y?=w765:bool)
                  n299 = Variant To Data(Variant=w769, type=sgl 0.0) -> (data=w766:sgl)  [unwired: 1 in, 1 out]
                  n300 = Format Into String(format string="%#f", w766) -> (resulting string=w762:string)  [unwired: 2 in, 1 out]
                  n301 = case shown="True" w765 {
                    tunnel: w761 -> [w774 w779]
                    tunnel: w763 -> [w771 _]
                    tunnel: w762 -> [w773 w782]
                    tunnel: [w772 w783] -> w760
                    frame False {
                      w777 = ">" ("string")
                      n302 = call <vilib>:"Space Constant.vi"() -> ("String"=w778:string)
                      n303 = Concatenate Strings("<" ("string"), w774, w778, w771, w777, w773, "</" ("string"), w774, w777) -> (w772:string)
                    }
                    frame True {
                      w780 = ">" ("string")
                      n304 = Concatenate Strings("<" ("string"), w779, w780, w782, "</" ("string"), w779, w780) -> (w783:string)
                    }
                  }
                }
                frame "Double Float" {
                  n305 = Get Variant Attribute(Variant=w793, name=w786) -> (duplicate Variant=w794:variant)  [unwired: 2 in, 3 out]
                  n306 = Equal?(x=w788, y="") -> (x = y?=w790:bool)
                  n307 = Variant To Data(Variant=w794, type=0.0) -> (data=w791:dbl)  [unwired: 1 in, 1 out]
                  n308 = Format Into String(format string="%#f", w791) -> (resulting string=w787:string)  [unwired: 2 in, 1 out]
                  n309 = case shown="True" w790 {
                    tunnel: w786 -> [w799 w804]
                    tunnel: w788 -> [w796 _]
                    tunnel: w787 -> [w798 w807]
                    tunnel: [w797 w808] -> w785
                    frame False {
                      w802 = ">" ("string")
                      n310 = call <vilib>:"Space Constant.vi"() -> ("String"=w803:string)
                      n311 = Concatenate Strings("<" ("string"), w799, w803, w796, w802, w798, "</" ("string"), w799, w802) -> (w797:string)
                    }
                    frame True {
                      w805 = ">" ("string")
                      n312 = Concatenate Strings("<" ("string"), w804, w805, w807, "</" ("string"), w804, w805) -> (w808:string)
                    }
                  }
                }
                frame "Extended Float" {
                  n313 = Get Variant Attribute(Variant=w818, name=w811) -> (duplicate Variant=w819:variant)  [unwired: 2 in, 3 out]
                  n314 = Equal?(x=w813, y="") -> (x = y?=w815:bool)
                  n315 = Variant To Data(Variant=w819, type=ext 0.0) -> (data=w816:ext)  [unwired: 1 in, 1 out]
                  n316 = Format Into String(format string="%#f", w816) -> (resulting string=w812:string)  [unwired: 2 in, 1 out]
                  n317 = case shown="True" w815 {
                    tunnel: w811 -> [w824 w829]
                    tunnel: w813 -> [w821 _]
                    tunnel: w812 -> [w823 w832]
                    tunnel: [w822 w833] -> w810
                    frame False {
                      w827 = ">" ("string")
                      n318 = call <vilib>:"Space Constant.vi"() -> ("String"=w828:string)
                      n319 = Concatenate Strings("<" ("string"), w824, w828, w821, w827, w823, "</" ("string"), w824, w827) -> (w822:string)
                    }
                    frame True {
                      w830 = ">" ("string")
                      n320 = Concatenate Strings("<" ("string"), w829, w830, w832, "</" ("string"), w829, w830) -> (w833:string)
                    }
                  }
                }
                frame "Single Complex" {
                  n321 = Get Variant Attribute(Variant=w841, name=w836) -> (duplicate Variant=w842:variant)  [unwired: 2 in, 3 out]
                  n322 = Equal?(x=w838, y="") -> (x = y?=w840:bool)
                  n323 = Variant To Data(Variant=w842, type=csg 0.0+0.0i ("number 3")) -> (data=w844:csg)  [unwired: 1 in, 1 out]
                  n324 = Format Value(value (0)=w844) -> (output string=w837:string)  [unwired: 2 in]
                  n325 = case shown="True" w840 {
                    tunnel: w836 -> [w848 w853]
                    tunnel: w838 -> [w845 _]
                    tunnel: w837 -> [w847 w856]
                    tunnel: [w846 w857] -> w835
                    frame False {
                      w851 = ">" ("string")
                      n326 = call <vilib>:"Space Constant.vi"() -> ("String"=w852:string)
                      n327 = Concatenate Strings("<" ("string"), w848, w852, w845, w851, w847, "</" ("string"), w848, w851) -> (w846:string)
                    }
                    frame True {
                      w854 = ">" ("string")
                      n328 = Concatenate Strings("<" ("string"), w853, w854, w856, "</" ("string"), w853, w854) -> (w857:string)
                    }
                  }
                }
                frame "Double Complex" {
                  n329 = Get Variant Attribute(Variant=w865, name=w860) -> (duplicate Variant=w866:variant)  [unwired: 2 in, 3 out]
                  n330 = Equal?(x=w862, y="") -> (x = y?=w864:bool)
                  n331 = Variant To Data(Variant=w866, type=cdb 0.0+0.0i ("number 3")) -> (data=w868:cdb)  [unwired: 1 in, 1 out]
                  n332 = Format Value(value (0)=w868) -> (output string=w861:string)  [unwired: 2 in]
                  n333 = case shown="True" w864 {
                    tunnel: w860 -> [w872 w877]
                    tunnel: w862 -> [w869 _]
                    tunnel: w861 -> [w871 w880]
                    tunnel: [w870 w881] -> w859
                    frame False {
                      w875 = ">" ("string")
                      n334 = call <vilib>:"Space Constant.vi"() -> ("String"=w876:string)
                      n335 = Concatenate Strings("<" ("string"), w872, w876, w869, w875, w871, "</" ("string"), w872, w875) -> (w870:string)
                    }
                    frame True {
                      w878 = ">" ("string")
                      n336 = Concatenate Strings("<" ("string"), w877, w878, w880, "</" ("string"), w877, w878) -> (w881:string)
                    }
                  }
                }
                frame "Extended Complex" {
                  n337 = Get Variant Attribute(Variant=w889, name=w884) -> (duplicate Variant=w890:variant)  [unwired: 2 in, 3 out]
                  n338 = Equal?(x=w886, y="") -> (x = y?=w888:bool)
                  n339 = Variant To Data(Variant=w890, type=cxt 0.0+0.0i ("number 3")) -> (data=w891:cxt)  [unwired: 1 in, 1 out]
                  n340 = Format Value(value (0)=w891) -> (output string=w885:string)  [unwired: 2 in]
                  n341 = case shown="True" w888 {
                    tunnel: w884 -> [w896 w901]
                    tunnel: w886 -> [w893 _]
                    tunnel: w885 -> [w895 w904]
                    tunnel: [w894 w905] -> w883
                    frame False {
                      w899 = ">" ("string")
                      n342 = call <vilib>:"Space Constant.vi"() -> ("String"=w900:string)
                      n343 = Concatenate Strings("<" ("string"), w896, w900, w893, w899, w895, "</" ("string"), w896, w899) -> (w894:string)
                    }
                    frame True {
                      w902 = ">" ("string")
                      n344 = Concatenate Strings("<" ("string"), w901, w902, w904, "</" ("string"), w901, w902) -> (w905:string)
                    }
                  }
                }
                frame "Boolean" {
                  n345 = Get Variant Attribute(Variant=w913, name=w908) -> (duplicate Variant=w914:variant)  [unwired: 2 in, 3 out]
                  n346 = Equal?(x=w910, y="") -> (x = y?=w912:bool)
                  n347 = Variant To Data(Variant=w914, type=TRUE) -> (data=w917:bool)  [unwired: 1 in, 1 out]
                  n348 = Boolean To (0,1)(Boolean=w917) -> (0, 1=w915:i16)
                  n349 = Number To Decimal String(number=w915) -> (decimal integer string=w909:string)  [unwired: 1 in]
                  n350 = case shown="True" w912 {
                    tunnel: w908 -> [w921 w926]
                    tunnel: w910 -> [w918 _]
                    tunnel: w909 -> [w920 w929]
                    tunnel: [w919 w930] -> w907
                    frame False {
                      w924 = ">" ("string")
                      n351 = call <vilib>:"Space Constant.vi"() -> ("String"=w925:string)
                      n352 = Concatenate Strings("<" ("string"), w921, w925, w918, w924, w920, "</" ("string"), w921, w924) -> (w919:string)
                    }
                    frame True {
                      w927 = ">" ("string")
                      n353 = Concatenate Strings("<" ("string"), w926, w927, w929, "</" ("string"), w926, w927) -> (w930:string)
                    }
                  }
                }
                frame "Array" {
                  n354 = call <vilib>:"GetArrayInfo.vi"("Variant"=w938) -> ("ArrayElement"=w940:variant)  [unwired: 7 in, 3 out]
                  n355 = Equal?(x=w933, y="") -> (x = y?=w936:bool)
                  n356 = call <vilib>:"GetTypeInfo.vi"("Variant"=w940) -> ("Type Enum"=w939:T6)  [unwired: 6 in, 4 out]
                  n357 = case shown="\"Single Float\"" w939 {
                    tunnel: w938 -> [w961 w976 w989 w1005 w1020 w1037 w1052 w1069 w1084 w1101 w1120 w1137 w1153 w1169 w1187]
                    tunnel: [w956 w974 w987 w1003 w1021 w1035 w1053 w1067 w1086 w1102 w1118 w1135 w1151 w1167 w1183] -> w934
                    tunnel: w933 -> [w955 w971 w988 w1004 w1019 w1036 w1051 w1068 w1083 w1100 w1119 w1136 w1152 w1168 w1186]
                    frame "I8" {
                      n358 = Get Variant Attribute(Variant=w961, name=w955) -> (duplicate Variant=w960:variant)  [unwired: 2 in, 3 out]
                      n359 = Variant To Data(Variant=w960, type=u8[] [] ("Array")) -> (data=w958:u8[])  [unwired: 1 in, 1 out]
                      n360 = while {
                        tunnel: w958 -> [w970] mode=indexing
                        tunnel: w958 -> [w969]
                        shift-right: [w962] -> w956
                        shift-left: "" -> [w963]
                        i -> [w967]
                        stop <- w966 stop-if-true
                        n361 = Array Size(array=w969) -> (size(s)=w968:i32)
                        n362 = Number To Decimal String(number=w970) -> (decimal integer string=w965:string)  [unwired: 1 in]
                        n363 = call <vilib>:"Space Constant.vi"() -> ("String"=w964:string)
                        n364 = Equal?(x=w968, y=w967) -> (x = y?=w966:bool)
                        n365 = Concatenate Strings(w963, w965, w964) -> (w962:string)
                      }
                    }
                    frame "I16" {
                      n366 = Get Variant Attribute(Variant=w976, name=w971) -> (duplicate Variant=w973:variant)  [unwired: 2 in, 3 out]
                      n367 = Variant To Data(Variant=w973, type=i16[] [] ("Array")) -> (data=w972:i16[])  [unwired: 1 in, 1 out]
                      n368 = while {
                        tunnel: w972 -> [w986] mode=indexing
                        shift-right: [w979] -> w974
                        shift-left: "" -> [w980]
                        tunnel: w972 -> [w978]
                        i -> [w984]
                        stop <- w983 stop-if-true
                        n369 = Array Size(array=w978) -> (size(s)=w985:i32)
                        n370 = Number To Decimal String(number=w986) -> (decimal integer string=w982:string)  [unwired: 1 in]
                        n371 = call <vilib>:"Space Constant.vi"() -> ("String"=w981:string)
                        n372 = Equal?(x=w985, y=w984) -> (x = y?=w983:bool)
                        n373 = Concatenate Strings(w980, w982, w981) -> (w979:string)
                      }
                    }
                    frame "I32" {
                      n374 = Get Variant Attribute(Variant=w989, name=w988) -> (duplicate Variant=w991:variant)  [unwired: 2 in, 3 out]
                      n375 = Variant To Data(Variant=w991, type=i16[] [] ("Array")) -> (data=w990:i16[])  [unwired: 1 in, 1 out]
                      n376 = while {
                        tunnel: w990 -> [w1002] mode=indexing
                        shift-right: [w995] -> w987
                        shift-left: "" -> [w996]
                        tunnel: w990 -> [w994]
                        i -> [w1000]
                        stop <- w999 stop-if-true
                        n377 = Array Size(array=w994) -> (size(s)=w1001:i32)
                        n378 = Number To Decimal String(number=w1002) -> (decimal integer string=w998:string)  [unwired: 1 in]
                        n379 = call <vilib>:"Space Constant.vi"() -> ("String"=w997:string)
                        n380 = Equal?(x=w1001, y=w1000) -> (x = y?=w999:bool)
                        n381 = Concatenate Strings(w996, w998, w997) -> (w995:string)
                      }
                    }
                    frame "I64" {
                      n382 = Get Variant Attribute(Variant=w1005, name=w1004) -> (duplicate Variant=w1007:variant)  [unwired: 2 in, 3 out]
                      n383 = Variant To Data(Variant=w1007, type=i64[] [] ("Array")) -> (data=w1006:i64[])  [unwired: 1 in, 1 out]
                      n384 = while {
                        tunnel: w1006 -> [w1018] mode=indexing
                        shift-right: [w1011] -> w1003
                        shift-left: "" -> [w1012]
                        tunnel: w1006 -> [w1010]
                        i -> [w1016]
                        stop <- w1015 stop-if-true
                        n385 = Array Size(array=w1010) -> (size(s)=w1017:i32)
                        n386 = Number To Decimal String(number=w1018) -> (decimal integer string=w1014:string)  [unwired: 1 in]
                        n387 = call <vilib>:"Space Constant.vi"() -> ("String"=w1013:string)
                        n388 = Equal?(x=w1017, y=w1016) -> (x = y?=w1015:bool)
                        n389 = Concatenate Strings(w1012, w1014, w1013) -> (w1011:string)
                      }
                    }
                    frame "U8" {
                      n390 = Get Variant Attribute(Variant=w1020, name=w1019) -> (duplicate Variant=w1023:variant)  [unwired: 2 in, 3 out]
                      n391 = Variant To Data(Variant=w1023, type=u8[] [] ("Array")) -> (data=w1022:u8[])  [unwired: 1 in, 1 out]
                      n392 = while {
                        tunnel: w1022 -> [w1034] mode=indexing
                        shift-right: [w1027] -> w1021
                        shift-left: "" -> [w1028]
                        tunnel: w1022 -> [w1026]
                        i -> [w1032]
                        stop <- w1031 stop-if-true
                        n393 = Array Size(array=w1026) -> (size(s)=w1033:i32)
                        n394 = Number To Decimal String(number=w1034) -> (decimal integer string=w1030:string)  [unwired: 1 in]
                        n395 = call <vilib>:"Space Constant.vi"() -> ("String"=w1029:string)
                        n396 = Equal?(x=w1033, y=w1032) -> (x = y?=w1031:bool)
                        n397 = Concatenate Strings(w1028, w1030, w1029) -> (w1027:string)
                      }
                    }
                    frame "U16" {
                      n398 = Get Variant Attribute(Variant=w1037, name=w1036) -> (duplicate Variant=w1039:variant)  [unwired: 2 in, 3 out]
                      n399 = Variant To Data(Variant=w1039, type=u16[] [] ("Array")) -> (data=w1038:u16[])  [unwired: 1 in, 1 out]
                      n400 = while {
                        tunnel: w1038 -> [w1050] mode=indexing
                        shift-right: [w1043] -> w1035
                        shift-left: "" -> [w1044]
                        tunnel: w1038 -> [w1042]
                        i -> [w1048]
                        stop <- w1047 stop-if-true
                        n401 = Array Size(array=w1042) -> (size(s)=w1049:i32)
                        n402 = Number To Decimal String(number=w1050) -> (decimal integer string=w1046:string)  [unwired: 1 in]
                        n403 = call <vilib>:"Space Constant.vi"() -> ("String"=w1045:string)
                        n404 = Equal?(x=w1049, y=w1048) -> (x = y?=w1047:bool)
                        n405 = Concatenate Strings(w1044, w1046, w1045) -> (w1043:string)
                      }
                    }
                    frame "U32" {
                      n406 = Get Variant Attribute(Variant=w1052, name=w1051) -> (duplicate Variant=w1055:variant)  [unwired: 2 in, 3 out]
                      n407 = Variant To Data(Variant=w1055, type=u32[] [] ("Array")) -> (data=w1054:u32[])  [unwired: 1 in, 1 out]
                      n408 = while {
                        tunnel: w1054 -> [w1066] mode=indexing
                        shift-right: [w1059] -> w1053
                        shift-left: "" -> [w1060]
                        tunnel: w1054 -> [w1058]
                        i -> [w1064]
                        stop <- w1063 stop-if-true
                        n409 = Array Size(array=w1058) -> (size(s)=w1065:i32)
                        n410 = Number To Decimal String(number=w1066) -> (decimal integer string=w1062:string)  [unwired: 1 in]
                        n411 = call <vilib>:"Space Constant.vi"() -> ("String"=w1061:string)
                        n412 = Equal?(x=w1065, y=w1064) -> (x = y?=w1063:bool)
                        n413 = Concatenate Strings(w1060, w1062, w1061) -> (w1059:string)
                      }
                    }
                    frame "U64" {
                      n414 = Get Variant Attribute(Variant=w1069, name=w1068) -> (duplicate Variant=w1071:variant)  [unwired: 2 in, 3 out]
                      n415 = Variant To Data(Variant=w1071, type=u64[] [] ("Array")) -> (data=w1070:u64[])  [unwired: 1 in, 1 out]
                      n416 = while {
                        tunnel: w1070 -> [w1082] mode=indexing
                        shift-right: [w1075] -> w1067
                        shift-left: "" -> [w1076]
                        tunnel: w1070 -> [w1074]
                        i -> [w1080]
                        stop <- w1079 stop-if-true
                        n417 = Array Size(array=w1074) -> (size(s)=w1081:i32)
                        n418 = Number To Decimal String(number=w1082) -> (decimal integer string=w1078:string)  [unwired: 1 in]
                        n419 = call <vilib>:"Space Constant.vi"() -> ("String"=w1077:string)
                        n420 = Equal?(x=w1081, y=w1080) -> (x = y?=w1079:bool)
                        n421 = Concatenate Strings(w1076, w1078, w1077) -> (w1075:string)
                      }
                    }
                    frame "Single Float" {
                      n422 = Get Variant Attribute(Variant=w1084, name=w1083) -> (duplicate Variant=w1087:variant)  [unwired: 2 in, 3 out]
                      n423 = Variant To Data(Variant=w1087, type=sgl[] [] ("Array")) -> (data=w1085:sgl[])  [unwired: 1 in, 1 out]
                      n424 = while {
                        tunnel: w1085 -> [w1091] mode=indexing
                        shift-right: [w1094] -> w1086
                        shift-left: "" -> [w1095]
                        tunnel: w1085 -> [w1093]
                        i -> [w1098]
                        stop <- w1097 stop-if-true
                        n425 = Array Size(array=w1093) -> (size(s)=w1099:i32)
                        n426 = Format Into String(format string="%#f", w1091) -> (resulting string=w1090:string)  [unwired: 2 in, 1 out]
                        n427 = Equal?(x=w1099, y=w1098) -> (x = y?=w1097:bool)
                        n428 = call <vilib>:"Space Constant.vi"() -> ("String"=w1096:string)
                        n429 = Concatenate Strings(w1095, w1090, w1096) -> (w1094:string)
                      }
                    }
                    frame "Double Float" {
                      n430 = Get Variant Attribute(Variant=w1101, name=w1100) -> (duplicate Variant=w1104:variant)  [unwired: 2 in, 3 out]
                      n431 = Variant To Data(Variant=w1104, type=dbl[] [] ("Array")) -> (data=w1103:dbl[])  [unwired: 1 in, 1 out]
                      n432 = while {
                        tunnel: w1103 -> [w1111] mode=indexing
                        shift-right: [w1114] -> w1102
                        shift-left: "" -> [w1115]
                        tunnel: w1103 -> [w1113]
                        i -> [w1107]
                        stop <- w1117 stop-if-true
                        n433 = Array Size(array=w1113) -> (size(s)=w1108:i32)
                        n434 = Format Into String(format string="%f", w1111) -> (resulting string=w1110:string)  [unwired: 2 in, 1 out]
                        n435 = Decrement(x=w1108) -> (x-1=w1109:i32)
                        n436 = Equal?(x=w1109, y=w1107) -> (x = y?=w1117:bool)
                        n437 = call <vilib>:"Space Constant.vi"() -> ("String"=w1116:string)
                        n438 = Concatenate Strings(w1115, w1110, w1116) -> (w1114:string)
                      }
                    }
                    frame "Extended Float" {
                      n439 = Get Variant Attribute(Variant=w1120, name=w1119) -> (duplicate Variant=w1122:variant)  [unwired: 2 in, 3 out]
                      n440 = Variant To Data(Variant=w1122, type=ext[] [] ("Array")) -> (data=w1121:ext[])  [unwired: 1 in, 1 out]
                      n441 = while {
                        tunnel: w1121 -> [w1126] mode=indexing
                        shift-right: [w1129] -> w1118
                        shift-left: "" -> [w1130]
                        tunnel: w1121 -> [w1128]
                        i -> [w1133]
                        stop <- w1132 stop-if-true
                        n442 = Array Size(array=w1128) -> (size(s)=w1134:i32)
                        n443 = Format Into String(format string="%#f", w1126) -> (resulting string=w1125:string)  [unwired: 2 in, 1 out]
                        n444 = Equal?(x=w1134, y=w1133) -> (x = y?=w1132:bool)
                        n445 = call <vilib>:"Space Constant.vi"() -> ("String"=w1131:string)
                        n446 = Concatenate Strings(w1130, w1125, w1131) -> (w1129:string)
                      }
                    }
                    frame "Single Complex" {
                      n447 = Get Variant Attribute(Variant=w1137, name=w1136) -> (duplicate Variant=w1139:variant)  [unwired: 2 in, 3 out]
                      n448 = Variant To Data(Variant=w1139, type=csg[] [] ("Array")) -> (data=w1138:csg[])  [unwired: 1 in, 1 out]
                      n449 = while {
                        tunnel: w1138 -> [w1143] mode=indexing
                        shift-right: [w1145] -> w1135
                        shift-left: "" -> [w1146]
                        tunnel: w1138 -> [w1144]
                        i -> [w1149]
                        stop <- w1148 stop-if-true
                        n450 = Array Size(array=w1144) -> (size(s)=w1150:i32)
                        n451 = Format Value(value (0)=w1143) -> (output string=w1142:string)  [unwired: 2 in]
                        n452 = call <vilib>:"Space Constant.vi"() -> ("String"=w1147:string)
                        n453 = Equal?(x=w1150, y=w1149) -> (x = y?=w1148:bool)
                        n454 = Concatenate Strings(w1146, w1142, w1147) -> (w1145:string)
                      }
                    }
                    frame "Double Complex" {
                      n455 = Get Variant Attribute(Variant=w1153, name=w1152) -> (duplicate Variant=w1155:variant)  [unwired: 2 in, 3 out]
                      n456 = Variant To Data(Variant=w1155, type=cdb[] [] ("Array")) -> (data=w1154:cdb[])  [unwired: 1 in, 1 out]
                      n457 = while {
                        tunnel: w1154 -> [w1159] mode=indexing
                        shift-right: [w1161] -> w1151
                        shift-left: "" -> [w1162]
                        tunnel: w1154 -> [w1160]
                        i -> [w1165]
                        stop <- w1164 stop-if-true
                        n458 = Array Size(array=w1160) -> (size(s)=w1166:i32)
                        n459 = Format Value(value (0)=w1159) -> (output string=w1158:string)  [unwired: 2 in]
                        n460 = call <vilib>:"Space Constant.vi"() -> ("String"=w1163:string)
                        n461 = Equal?(x=w1166, y=w1165) -> (x = y?=w1164:bool)
                        n462 = Concatenate Strings(w1162, w1158, w1163) -> (w1161:string)
                      }
                    }
                    frame "Extended Complex" {
                      n463 = Get Variant Attribute(Variant=w1169, name=w1168) -> (duplicate Variant=w1171:variant)  [unwired: 2 in, 3 out]
                      n464 = Variant To Data(Variant=w1171, type=cxt[] [] ("Array")) -> (data=w1170:cxt[])  [unwired: 1 in, 1 out]
                      n465 = while {
                        tunnel: w1170 -> [w1175] mode=indexing
                        shift-right: [w1177] -> w1167
                        shift-left: "" -> [w1178]
                        tunnel: w1170 -> [w1176]
                        i -> [w1181]
                        stop <- w1180 stop-if-true
                        n466 = Array Size(array=w1176) -> (size(s)=w1182:i32)
                        n467 = Format Value(value (0)=w1175) -> (output string=w1174:string)  [unwired: 2 in]
                        n468 = call <vilib>:"Space Constant.vi"() -> ("String"=w1179:string)
                        n469 = Equal?(x=w1182, y=w1181) -> (x = y?=w1180:bool)
                        n470 = Concatenate Strings(w1178, w1174, w1179) -> (w1177:string)
                      }
                    }
                    frame "String", Default {
                      n471 = Get Variant Attribute(Variant=w1187, name=w1186) -> (duplicate Variant=w1188:variant)  [unwired: 2 in, 3 out]
                      n472 = Variant To Data(Variant=w1188, type=string[] [] ("Array")) -> (data=w1184:string[])  [unwired: 1 in, 1 out]
                      n473 = while {
                        tunnel: w1184 -> [w1190] mode=indexing
                        shift-right: [w1192] -> w1183
                        shift-left: "" -> [w1193]
                        tunnel: w1184 -> [w1191]
                        i -> [w1196]
                        stop <- w1195 stop-if-true
                        n474 = call <vilib>:"Space Constant.vi"() -> ("String"=w1194:string)
                        n475 = Array Size(array=w1191) -> (size(s)=w1197:i32)
                        n476 = Concatenate Strings(w1193, w1190, w1194) -> (w1192:string)
                        n477 = Equal?(x=w1197, y=w1196) -> (x = y?=w1195:bool)
                      }
                    }
                  }
                  n478 = case shown="False" w936 {
                    tunnel: w933 -> [w944 w949]
                    tunnel: w932 -> [w941 _]
                    tunnel: w934 -> [w943 w952]
                    tunnel: [w942 w953] -> w937
                    frame False {
                      w947 = ">" ("string")
                      n479 = call <vilib>:"Space Constant.vi"() -> ("String"=w948:string)
                      n480 = Concatenate Strings("<" ("string"), w944, w948, w941, w947, w943, "</" ("string"), w944, w947) -> (w942:string)
                    }
                    frame True {
                      w950 = ">" ("string")
                      n481 = Concatenate Strings("<" ("string"), w949, w950, w952, "</" ("string"), w949, w950) -> (w953:string)
                    }
                  }
                }
                frame "String", Default {
                  n482 = Get Variant Attribute(Variant=w1204, name=w1202) -> (duplicate Variant=w1205:variant)  [unwired: 2 in, 3 out]
                  n483 = Equal?(x=w1200, y="") -> (x = y?=w1201:bool)
                  n484 = Variant To Data(Variant=w1205, type="") -> (data=w1203:string)  [unwired: 1 in, 1 out]
                  n485 = case shown="True" w1201 {
                    tunnel: w1202 -> [w1210 w1215]
                    tunnel: w1200 -> [w1207 _]
                    tunnel: w1203 -> [w1209 w1218]
                    tunnel: [w1208 w1219] -> w1198
                    frame False {
                      w1213 = ">" ("string")
                      n486 = call <vilib>:"Space Constant.vi"() -> ("String"=w1214:string)
                      n487 = Concatenate Strings("<" ("string"), w1210, w1214, w1207, w1213, w1209, "</" ("string"), w1210, w1213) -> (w1208:string)
                    }
                    frame True {
                      w1216 = ">" ("string")
                      n488 = Concatenate Strings("<" ("string"), w1215, w1216, w1218, "</" ("string"), w1215, w1216) -> (w1219:string)
                    }
                  }
                }
                frame "Fixed Point" {
                  n489 = Get Variant Attribute(Variant=w1230, name=w1222) -> (duplicate Variant=w1231:variant)  [unwired: 2 in, 3 out]
                  n490 = Equal?(x=w1224, y="") -> (x = y?=w1226:bool)
                  n491 = Variant To Data(Variant=w1231, type=fxp<+,1,1> 0.0) -> (data=w1228:fxp<+,1,1>)  [unwired: 1 in, 1 out]
                  n492 = Format Into String(format string="%#f", w1228) -> (resulting string=w1223:string)  [unwired: 2 in, 1 out]
                  n493 = case shown="True" w1226 {
                    tunnel: w1222 -> [w1235 w1240]
                    tunnel: w1224 -> [w1232 _]
                    tunnel: w1223 -> [w1234 w1243]
                    tunnel: [w1233 w1244] -> w1221
                    frame False {
                      w1238 = ">" ("string")
                      n494 = call <vilib>:"Space Constant.vi"() -> ("String"=w1239:string)
                      n495 = Concatenate Strings("<" ("string"), w1235, w1239, w1232, w1238, w1234, "</" ("string"), w1235, w1238) -> (w1233:string)
                    }
                    frame True {
                      w1241 = ">" ("string")
                      n496 = Concatenate Strings("<" ("string"), w1240, w1241, w1243, "</" ("string"), w1240, w1241) -> (w1244:string)
                    }
                  }
                }
              }
            }
            n497 = Concatenate Strings(w556, w558, w555) -> (w559:string)
            n498 = local write "XML-String-out"(w559) -> ()
          }
          frame "Set" {
            n499 = local read "error in (no error)"() -> (→"error in (no error) 2":errorcluster)
            n500 = local read "Database"() -> (w1260:string)
            n501 = local read "XML-String-out"() -> (w1254:string)
            n502 = Wait (ms)(milliseconds to wait=u32 1000) -> ()  [unwired: 1 out]
            n503 = call-poly <vilib>:"DB Tools Open Connection.vi"("error in (no error)"=errorcluster {"status"=FALSE, "code"=0, "source"=""}, "connection information"=w1260) -> ("error out"=w1248:errorcluster, "connection reference"=w1252:T4)  [unwired: 6 in]
            n504 = Unbundle By Name(w1248) -> ("status"=w1257:bool, "code"=w1251:i32, "source"=w1255:string)
            n505 = local read "exp_id"() -> (w1253:i32)
            n506 = case shown="True" w1257 {
              selector: w1257 -> [w1301 _]
              tunnel: w1251 -> [w1300 _]
              tunnel: w1255 -> [w1278 w1324]
              tunnel: [w1299 errorcluster {"status"=FALSE, "code"=0, "source"=""} ("error in (no error)")] -> w1249
              tunnel: w1252 -> [w1298 w1337]
              tunnel: [w1296 w1328] -> w1250
              tunnel: w1254 -> [w1288 w1336]
              tunnel: w1253 -> [w1287 w1335]
              frame False {
                w1262 = "' WHERE exp_id =" ("string")
                w1280 = "\t"
                w1263 = " WHERE exp_id ="
                n507 = Get Date/Time In Seconds() -> (seconds since 1Jan1904=w1270:timestamp)
                n508 = local read "submit_time"() -> (w1267:timestamp)
                n509 = local read "exec_time"() -> (w1268:timestamp)
                n510 = Subtract(x=w1270, y=w1268) -> (x-y=w1276:dbl)
                n511 = Subtract(x=w1270, y=w1267) -> (x-y=w1275:dbl)
                n512 = Number To Decimal String(number=w1287) -> (decimal integer string=w1271:string)  [unwired: 1 in]
                n513 = Format Date/Time String(seconds (now)=w1270) -> (date/time string=w1281:string)  [unwired: 2 in]
                n514 = local read "Status"() -> (w1285:string)
                n515 = To Long Integer(number=w1276) -> (32bit integer=w1265:i32)
                n516 = To Long Integer(number=w1275) -> (32bit integer=w1264:i32)
                n517 = Format Date/Time String(seconds (now)=w1270) -> (date/time string=w1291:string)  [unwired: 2 in]
                n518 = Number To Decimal String(number=w1265) -> (decimal integer string=w1269:string)  [unwired: 1 in]
                n519 = Number To Decimal String(number=w1264) -> (decimal integer string=w1273:string)  [unwired: 1 in]
                n520 = Concatenate Strings(w1285, "Job completed!! exp_id = " ("string"), w1271, w1280, w1280, w1281, "\r\n") -> (w1284:string)
                n521 = Concatenate Strings("UPDATE dbo.JobRecord SET end_time = '", w1291, w1262, w1271) -> (w1295:string)
                n522 = Concatenate Strings("UPDATE dbo.JobRecord SET error_report = '" ("string"), w1278, w1262, w1271) -> (w1277:string)
                n523 = Concatenate Strings("UPDATE dbo.JobRecord SET exec_elapsed = ", w1269, w1263, w1271) -> (w1266:string)
                n524 = Concatenate Strings("UPDATE dbo.JobRecord SET job_elapsed = ", w1273, w1263, w1271) -> (w1261:string)
                n525 = local write "Status"(w1284) -> ()
                n526 = Concatenate Strings("UPDATE dbo.JobRecord SET experiment_results = '", w1288, w1262, w1271) -> (w1293:string)
                n527 = Concatenate Strings("UPDATE dbo.JobRecord SET job_status = 'COMPLETE' WHERE exp_id =", w1271) -> (w1294:string)
                n528 = Concatenate Strings(w1293, w1294, w1295, w1277, w1266, w1261) -> (w1286:string)
                n529 = call-poly <vilib>:"DB Tools Execute Query.vi"("SQL query"=w1286, "connection reference"=w1298) -> ("recordset reference"=w1297:T5)  [unwired: 6 in, 1 out]
                n530 = call-poly <vilib>:"DB Tools Free Object.vi"("recordset reference"=w1297) -> ("connection reference"=w1296:T4)  [unwired: 9 in, 1 out]
                n531 = Bundle(w1301, "code"=w1300, "source"=w1278) -> (w1299:cluster{bool, "code":i32, "source":string})  [unwired: 1 in]
              }
              frame True {
                w1303 = "WHERE exp_id =" ("string")
                w1322 = "\t"
                w1307 = "' WHERE exp_id ="
                n532 = Get Date/Time In Seconds() -> (seconds since 1Jan1904=w1312:timestamp)
                n533 = local read "submit_time"() -> (w1311:timestamp)
                n534 = local read "exec_time"() -> (w1321:timestamp)
                n535 = Format Date/Time String(seconds (now)=w1312) -> (date/time string=w1319:string)  [unwired: 2 in]
                n536 = Number To Decimal String(number=w1335) -> (decimal integer string=w1306:string)  [unwired: 1 in]
                n537 = Subtract(x=w1312, y=w1321) -> (x-y=w1316:dbl)
                n538 = Subtract(x=w1312, y=w1311) -> (x-y=w1310:dbl)
                n539 = local read "Status"() -> (w1326:string)
                n540 = call <vilib>:"Space Constant.vi"() -> ("String"=w1317:string)
                n541 = To Long Integer(number=w1316) -> (32bit integer=w1304:i32)
                n542 = To Long Integer(number=w1310) -> (32bit integer=w1305:i32)
                n543 = Concatenate Strings(w1326, "Error occurred: " ("Status"), w1324, "exp_id = " ("string"), w1306, w1322, w1322, w1317, w1319, "\r\n") -> (w1325:string)
                n544 = Number To Decimal String(number=w1305) -> (decimal integer string=w1308:string)  [unwired: 1 in]
                n545 = local write "Status"(w1325) -> ()
                n546 = Format Date/Time String(seconds (now)=w1312) -> (date/time string=w1318:string)  [unwired: 2 in]
                n547 = Number To Decimal String(number=w1304) -> (decimal integer string=w1314:string)  [unwired: 1 in]
                n548 = Concatenate Strings("UPDATE dbo.JobRecord SET error_report = '" ("string"), w1324, w1307, w1306) -> (w1330:string)
                n549 = Concatenate Strings("UPDATE dbo.JobRecord SET end_time = '", w1317, w1318, w1307, w1306) -> (w1332:string)
                n550 = Concatenate Strings("UPDATE dbo.JobRecord SET exec_elapsed = ", w1314, w1303, w1306) -> (w1313:string)
                n551 = Concatenate Strings("UPDATE dbo.JobRecord SET job_elapsed = ", w1308, w1303, w1306) -> (w1302:string)
                n552 = Concatenate Strings("UPDATE dbo.JobRecord SET experiment_results = '", w1336, w1307, w1306) -> (w1342:string)
                n553 = Concatenate Strings("UPDATE dbo.JobRecord SET job_status = 'IN PROGRESS' WHERE exp_id =", w1306) -> (w1343:string)
                n554 = Concatenate Strings("UPDATE dbo.JobRecord SET error_occurred = 'True' WHERE epx_id =  " ("string"), w1306) -> (w1333:string)
                n555 = Concatenate Strings(w1342, w1343, w1333, w1330, w1332, w1313, w1302) -> (w1338:string)
                n556 = call-poly <vilib>:"DB Tools Execute Query.vi"("SQL query"=w1338, "connection reference"=w1337) -> ("error out"=w1329:errorcluster, "recordset reference"=w1344:T5)  [unwired: 6 in]
                n557 = call-poly <vilib>:"DB Tools Free Object.vi"("error in (no error)"=w1329, "recordset reference"=w1344) -> ("connection reference"=w1328:T4)  [unwired: 8 in, 1 out]
              }
            }
            n558 = call <vilib>:"DB Tools Close Connection.vi"("error in (no error)"=w1249, "connection reference"=w1250) -> ("error out"=w1256:errorcluster)  [unwired: 5 in]
            n559 = local write "error in (no error)"(w1256) -> ()
          }
        }
        n560 = case shown="True" "Stop" {
          selector: "Stop" -> [w39 w40]
          tunnel: [w39 w40] -> w34
          frame False {
          }
          frame True {
            n561 = invoke on="Indicator TAG" class="Str" method="Reinit To Default"() -> ()  [unwired: 3 in, 3 out]
            n562 = invoke on="Control TAG" class="Str" method="Reinit To Default"() -> ()  [unwired: 3 in, 3 out]
            n563 = invoke on="Experiment VI" class="Str" method="Reinit To Default"() -> ()  [unwired: 3 in, 3 out]
            n564 = invoke on="Stop" class="Bool (strict)" method="Reinit To Default"() -> ()  [unwired: 3 in, 3 out]
            n565 = invoke on="Status" class="Str" method="Reinit To Default"() -> ()  [unwired: 3 in, 3 out]
            n566 = invoke on="Result: XML Header" class="Str" method="Reinit To Default"() -> ()  [unwired: 3 in, 3 out]
            n567 = invoke on="Result: XML Footer" class="Str" method="Reinit To Default"() -> ()  [unwired: 3 in, 3 out]
            n568 = invoke on="Database" class="Str" method="Reinit To Default"() -> ()  [unwired: 3 in, 3 out]
          }
        }
        n569 = property on="Status" class="Str"("Text.Scroll Position"=inf) -> ()  [unwired: 2 in, 2 out]
      }
    }
  }
